vi "Dashboard Main.vi"() -> ()   [LabVIEW 2018]
uses:
  <vilib>/Utility/miscctls.llb/LVRowAndColumnTypeDef.ctl
  <vilib>/event_ctls.llb/eventvkey.ctl
  <vilib>/Rock Robotics/Network Tables/NT Read Numeric Array.vi
  <vilib>/Rock Robotics/Network Tables/NT Read Boolean.vi
  <vilib>/Rock Robotics/Network Tables/NT Write Boolean.vi
  <vilib>/Rock Robotics/WPI/Dashboard/WPI_DashboardLogging Global.vi
  <vilib>/Utility/xml.llb/Read From XML File(array).vi
  <vilib>/Utility/xml.llb/Write to XML File(string).vi
  <vilib>/vision/NI_Vision_Development_Module.lvlib
panel:
  out "Camera Image1":T1(plugin-control)
  out "Camera Image Right":T1(plugin-control)
  in  "Camera Settings Right":T2={"Frame Rate"=30, "Compression"=30, "Size"=1, "DB Camera Config"=FALSE} {"Frame Rate" scale=1.0..30.0; "Compression" scale=100.0..-1.0; "Size" items=["640x480", "320x240", "160x120"]}
  in  "Camera Name Right":string(combo)="No Camera Selection"
  in  "TCP":refnum<k5>
  in  "Rec Mode":enum32{"Stop", "Record", "Playback"}(radio)
  out "Robot IP":string
  out "Image Message":string="Timeout in Camera Communications"
  in  "Dashboard Tab":T3(tab)=enum."TeleOp"
  in  "CheckList":i32(listbox)
  out "Ret_CARGO Center":bool
  out "Elevator_Motor_Failure_2":bool
  out "Elevator_Stall":bool
  out "Range_Color_Front-Right":u32(colorbox)
  in  "Right":bool
  in  "Reticule":T4(ring)
  in  "Save":bool
  in  "Up":bool
  in  "Down":bool
  in  "Left":bool
  out "Ret_HATCH Right":bool
  out "Ret_HATCH Left":bool
  out "Ret_CARGO Right":bool
  out "Ret_CARGO Left":bool
  out "Out_Of_Time":bool caption="Mode_Butterfly"
  out "Match Time(s)":sgl
  out "Intake_In":bool caption="Mode_Butterfly"
  in  "Climb_Safety":bool
  out "Master_Caution":bool caption="Mode_Butterfly"
  out "Climb_Sequence":string
  out "Range_to_Target (R)":i16(slide)=-100 scale=-10.0..-50.0
  out "Range_to_Target (L)":i16(slide)=-100 scale=-50.0..-10.0
  out "Tilt_Interlock":bool
  out "Battery_Critical":bool
  out "Battery_Voltage":dbl(slide) scale=11.0..13.0
  out "COM_Warning":bool
  out "Elevator_Moving":bool caption="Mode_Butterfly"
  out "Range_Color_Back":u32(colorbox)
  out "Range_Color_Front-Left":u32(colorbox)
  out "Range_Color_Right":u32(colorbox)
  out "Range_Color_Left":u32(colorbox)
  out "Hatch_Ship_Light":bool
  out "Hatch_Rocket_1_Light":bool
  out "Hatch_Ground_Light":bool
  out "Hatch_Feeder_Light":bool
  out "Hatch_Rocket_2_Light":bool
  out "Hatch_Rocket_3_Light":bool
  out "Pressure_Visualize":dbl(slide) scale=0.0..120.0
  out "Autopilot":bool caption="Mode_Butterfly"
  in  "Master_Safety_Override_1":bool
  in  "Master_Safety_Override_2":bool
  out "Climb_Light":bool
  out "At Climb_Height":bool caption="Mode_Butterfly"
  out "PTO_Engaged":bool caption="Mode_Butterfly"
  in  "Climb":bool
  out "Mode_Butterfly":bool
  out "Compressor_On":bool
  out "Hatch_Ejection_State":bool caption="Mode_Butterfly"
  out "Elevator_Brake_State":bool
  out "Mode_Shift":bool caption="Mode_Butterfly"
  out "Capture_Cargo":bool caption="Mode_Butterfly"
  out "Capture_Hatch":bool caption="Mode_Butterfly"
  out "Right Feed":T1(plugin-control)
  in  "Hatch_Ground":bool
  in  "Hatch_Feeder":bool
  in  "Hatch_Rocket_2":bool
  in  "Hatch_Rocket_1":bool
  in  "Hatch_Ship":bool
  in  "Hatch_Rocket_3":bool
  out "Elevator_Stow_Light":bool
  in  "Elevator_Stow":bool
  out "Cargo_Ground_Light":bool
  out "Cargo_Feeder_Light":bool
  out "Cargo_Ship_Light":bool
  out "Cargo_Rocket_3_Light":bool
  in  "Cargo_Ground":bool
  in  "Cargo_Feeder":bool
  out "Cargo_Rocket_2_Light":bool
  out "Cargo_Rocket_1_Light":bool
  in  "Cargo_Ship":bool
  in  "Cargo_Rocket_1":bool
  in  "Cargo_Rocket_2":bool
  in  "Cargo_Rocket_3":bool
  out "State_Conflict":bool caption="Mode_Butterfly"
  out "Left Feed":T1(plugin-control)
  out "Elevator_Pos_Visual":dbl(slide) scale=34.5..89.0
  in  "Vision_Target_L_R":bool
  out "Elevator_Goal_Visual":dbl(slide) scale=34.5..89.0
  out "Elevator_Power":dbl(knob) scale=-1.0..1.0
  in  "Climb_Level":u8(slide)=1 scale=0.0..2.0
  in  "Driver Profile":u16(ring) items=["N/A"]
  out "E1 Warning":bool
  out "E2 Warning":bool
  out "E3 Warning":bool
  out "Elevator_3_Current":dbl format="%.1g"
  out "Elevator_2_Current":dbl format="%.1g"
  out "Elevator_1_Current":dbl format="%.1g"
  out "Slow_Loop":bool
  in  "Camera Settings 2":T2={"Frame Rate"=20, "Compression"=60, "Size"=1, "DB Camera Config"=FALSE} {"Size" items=["640x480", "320x240", "160x120"]}
  in  "Elevator_Kf_1":dbl(slide)=0.16 min=0.0 max=1.0 scale=0.0..1.0
  in  "Elevator_Kf_2":dbl(slide)=0.16 min=0.0 max=1.0 scale=0.0..1.0
  in  "Elevator_Kf_3":dbl(slide) min=0.0 max=1.0 scale=0.0..1.0
  in  "Select Auto":string(combo)="Select Autonomous ..."
  out "Camera Perf":string
  in  "Elevator_Kf_Climb":dbl(slide)=0.1 min=0.0 max=1.0 scale=0.0..1.0
  out "Control Loop Time (ms)":u32
  in  "Vacuum_Pump":dbl(slide)=0.6 min=0.0 max=1.0 scale=0.0..1.0
  out "Range_Right":dbl format="%.1g"
  in  "Elevator_Manual":bool
  in  "Drive_Encoder_Reset":bool
  out "Right_Drive_Pos":dbl
  out "Left_Drive_Pos":dbl
  out "Range_Left":dbl format="%.1g"
  out "Range_Front-Left":dbl format="%.1g"
  out "Range_Front-Right":dbl format="%.1g"
  out "Left_Drive_Vel":dbl format="%.1g"
  out "Right_Drive_Vel":dbl format="%.1g"
  out "Elevator_Pos":dbl format="%.1g"
  out "Range_Back":dbl
  out "Tank_Pressure":dbl
  in  "Super_Test_Mode":bool
  out "Ground_Height":dbl format="%.1g"
  in  "Overclock":bool=TRUE
  in  "Reinit_Stow_Vacuum":bool
  in  "LimeLight_Override":bool
  out "Elevator_Encoder_Malfunction":bool
  in  "Warning Time (s)":dbl=30.0
  out "Elevator_Motor_Failure":bool
  out "Robot_On_Ground":bool=TRUE
  out "Robot_Off_Ground":bool
  out "Check_Limit_Switch":bool
  in  "Tilt_Safety_Override":bool
  in  "Defense_Driving":bool
  out "NT Connection":bool
  out "Mode":T5(ring)=enum."Auto Disabled"
  out "Right Camera Perf":cluster{"Bandwidth (Mbps)":dbl, "FPS":dbl}
  in  "Test Slider":dbl(slide) scale=0.0..100.0 scale format="%#_3g"
  in  "On/Off":bool caption="Solenoid"
  in  "Test Name":u16(ring) items=["Select the test to run..."]
  in  "Test Tree":string(tree)
  in  "Motor":cluster{"Value":dbl, "Enable":bool} {"Value" scale=-1.0..1.0 scale format="%#_3g"}
  out "Progress":T6 {"Test Progress" scale=0.0..100.0}
  in  "Rev/Fwd":cluster{"Forward":bool, "Reverse":bool}
  in  "Test Ring":u16(ring) items=["Monochrome", "Color"]
  out "Cmd Status":string
  in  "Execute Command":bool
  in  "Command Params":string[][](table)
  in  "Command Selection":i32(listbox)
  out "Tree":string(tree)
  out "Background":bool
  in  "Camera Name":string(combo)="IMAQdx:Microsoft LifeCam"
  # "HW"
  # "11"
  # "13"
  # "Tina"
  # "Control Loop (ms)"
  # "Elevator Feed Forward Coefficients"
  # "Drive Wheel Velocities (ft/s)"
  # "Manual Elevator Override"
  # "Tilt Interlock Off"
  # "Wide-Cam Override"
  # "Reinit.  Vacuum in Stow"
  # "Super Test Mode"
  # "Elevator Position (in)"
  # "Prox Sensors (in)"
  # "Auto Elevator"
  # "Safe"
  # "Vacuum \nPump Power"
  # "Normal"
  # "Normal"
  # "Safe"
  # "Stage 2"
  # "Stage 3"
  # "Climb"
  # "Ground Height (in)"
  # "Elevator Motor Currents (A)"
  # "On \nGround"
  # "Off\nGround"
  # "E1"
  # "E2"
  # "E3"
  # "Match End Warning (s)"
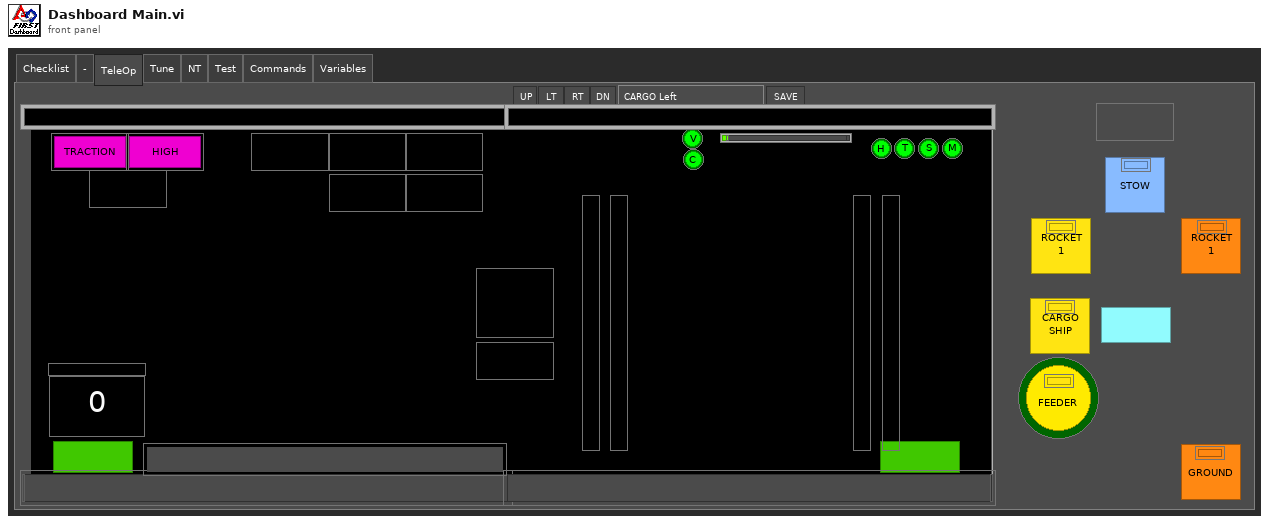
[diagram p1: front panel]
types:
  T1 = typedef "IMAQ Image.ctl" = refnum<image>
  T2 = cluster{"Frame Rate":i32, "Compression":i32, "Size":u16, "DB Camera Config":bool}
  T3 = enum32{"Checklist", "-", "TeleOp", "Tune", "NT", "Test", "Commands", "Variables"}
  T4 = enum16{"CARGO Left", "CARGO Right", "HATCH Left", "HATCH Right", "CARGO Center"}
  T5 = enum8{"Tele-Op Disabled", "Tele-Op Enabled", "Auto Disabled", "Auto Enabled", "Test Disabled", "Test Enabled", "Disconnected", "No Code", "E-Stop"}
  T6 = cluster{"Test Progress":u8, "Test Progress Text":string}
  T7 = cluster{"Save Path":path, "Interval (s)":dbl, "Keep":i32}
  T8 = enum32{"Drive", "Camera", "Basic", "Custom", "Test", "Commands", "Checklist", "Variables"}
  T9 = typedef "Image Type" = u32
  T10 = cluster{"IDs":cluster{"RPC field ID":u16, "Unique ID":u16}, "String":string}
  T11 = cluster{"Camera Image1":refnum<vi>, "Dashboard Tab":refnum<vi>, "Background":refnum<vi>, "Rec Mode":refnum<vi>, "Test Slider":refnum<vi>, "On/Off ":refnum<vi>, "Test Ring":refnum<vi>, "Rev/Fwd":refnum<vi>, "Test Name":refnum<vi>, "Motor":refnum<vi>, "Progress":refnum<vi>, "CheckList":refnum<vi>, "Tree":refnum<vi>, "Test Tree":refnum<vi>, "Command Params":refnum<vi>, "Command Selection":refnum<vi>, "Execute Command":refnum<vi>, "Cmd Status":refnum<vi>, "Camera Settings 2":refnum<vi>, "Camera Name":refnum<vi>, "Camera Perf":refnum<vi>, "Camera Settings Right":refnum<vi>, "Camera Name Right":refnum<vi>, "Camera Image Right":refnum<vi>}
  T12 = cluster{"Global Rectangle":i32[], "Contours":cluster{"Contour Type":u32, "ROI Type":u32, "Points":i32[]}[]}
  T13 = cluster{string, string, "Saved DB Images Info":cluster{"Save Path":path, "Interval (s)":dbl, "Keep":i32}}
  T14 = cluster{"Error Strings":string, "Disable Counts":cluster{u16, u16}, "Rail Faults":cluster{u16, u16, u16}, "Robot IP":string, "DB Mode":u8, "Event Info":cluster{"Name":string, "Type":u8, "Number":u16, "Replay":u8}}
  T15 = cluster{"Storage":cluster{"Disk Free":u64, "RAM Block":u32, "RAM free":u32}, "CPU Utilization":cluster{"CPU % ISR":sgl, "CPU % Time Crit":sgl, "CPU % Timed Str":sgl, "CPU % High":sgl, "CPU % Above":sgl, "CPU % Normal":sgl, "CPU % Low":sgl}, "CAN":cluster{"% Bus Utilization":sgl, "Bus Off Cnt":u32, "TX_FIFO Full Cnt":u32, "Receive Error Cnt":u8, "Transmit Error Cnt":u8}, "HID":cluster{"HID Outputs":u32, "Rumble Low":u16, "Rumble High":u16}[]}
  T16 = cluster{"Status bits":cluster{"Test Mode":bool, "Autonomous":bool, "Enabled":bool, "Code Start":bool, "Brownout":bool, "Reserved 2":bool, "Reserved 3":bool, "E-Stop":bool}, "Code Trace":cluster{"Disabled":bool, "TeleOp":bool, "Auto":bool, "Test":bool}, "Controller Type":enum16{"unknown", "cRIO", "roboRio"}, "Code?":enum16{"unknown", "noCode", "code"}, "Battery V":dbl}
  T17 = cluster{"Control Bits":cluster{"TestMode":bool, "Autonomous":bool, "Enabled":bool, "FMS Present":bool, bool, bool, bool, "E-Stop":bool}, "Team Station ":u8, "Countdown":sgl, "Joystick Values":cluster{"Axes":dbl[], "Buttons":bool[], "POVs":i16[]}[]}
  T18 = cluster{"Axes":dbl[], "Buttons":bool[], "POVs":i16[]}[]
  T19 = cluster{"Axes":dbl[], "Buttons":bool[], "POVs":i16[]}
  T20 = cluster{"Operation":enum16{"Update", "Clear"}, "Color Box":u32}[]
  T21 = typedef "eventvkey.ctl" = enum16{"ASCII", "Enter", "Return", "Shift", "Ctrl", "Alt", "Cmd", "Opt", "Caps", "NumLock", "Clear", "Break", "Up", "Down", "Left", "Right", "Insert", "Delete", "Home", "End", "PageUp", "PageDown", "Escape", "Help", "Pause", "ScrollLock", "F1", "F2", "F3", "F4", "F5", "F6", "F7", "F8", "F9", "F10", "F11", "F12", "F13", "F14", "F15", "F16", "F17", "F18", "F19", "F20", "F21", "F22", "F23", "F24", "Play", "VolumeUp", "VolumeDown", "Mute", "Two Byte Char"}
  T22 = cluster{"Image Size":bool, "Image Type":bool, "Pixel Value":bool, "ROI Information":bool, "Zoom Factor":bool}
  T23 = cluster{"Operation":enum16{"Update", "Clear"}, "Color Box":u32}
  T24 = typedef "LVRowAndColumnTypeDef.ctl" = cluster{"Row":i32, "Column":i32}
  T25 = cluster{"Shift":bool, "Ctrl":bool, "Alt":bool, "Cmd":bool, "Opt":bool}
  T26 = cluster{"Ret_CARGO Left":refnum<vi>, "Ret_CARGO Right":refnum<vi>, "Ret_HATCH Left":refnum<vi>, "Ret_HATCH Right":refnum<vi>, "Ret_CARGO Center":refnum<vi>}
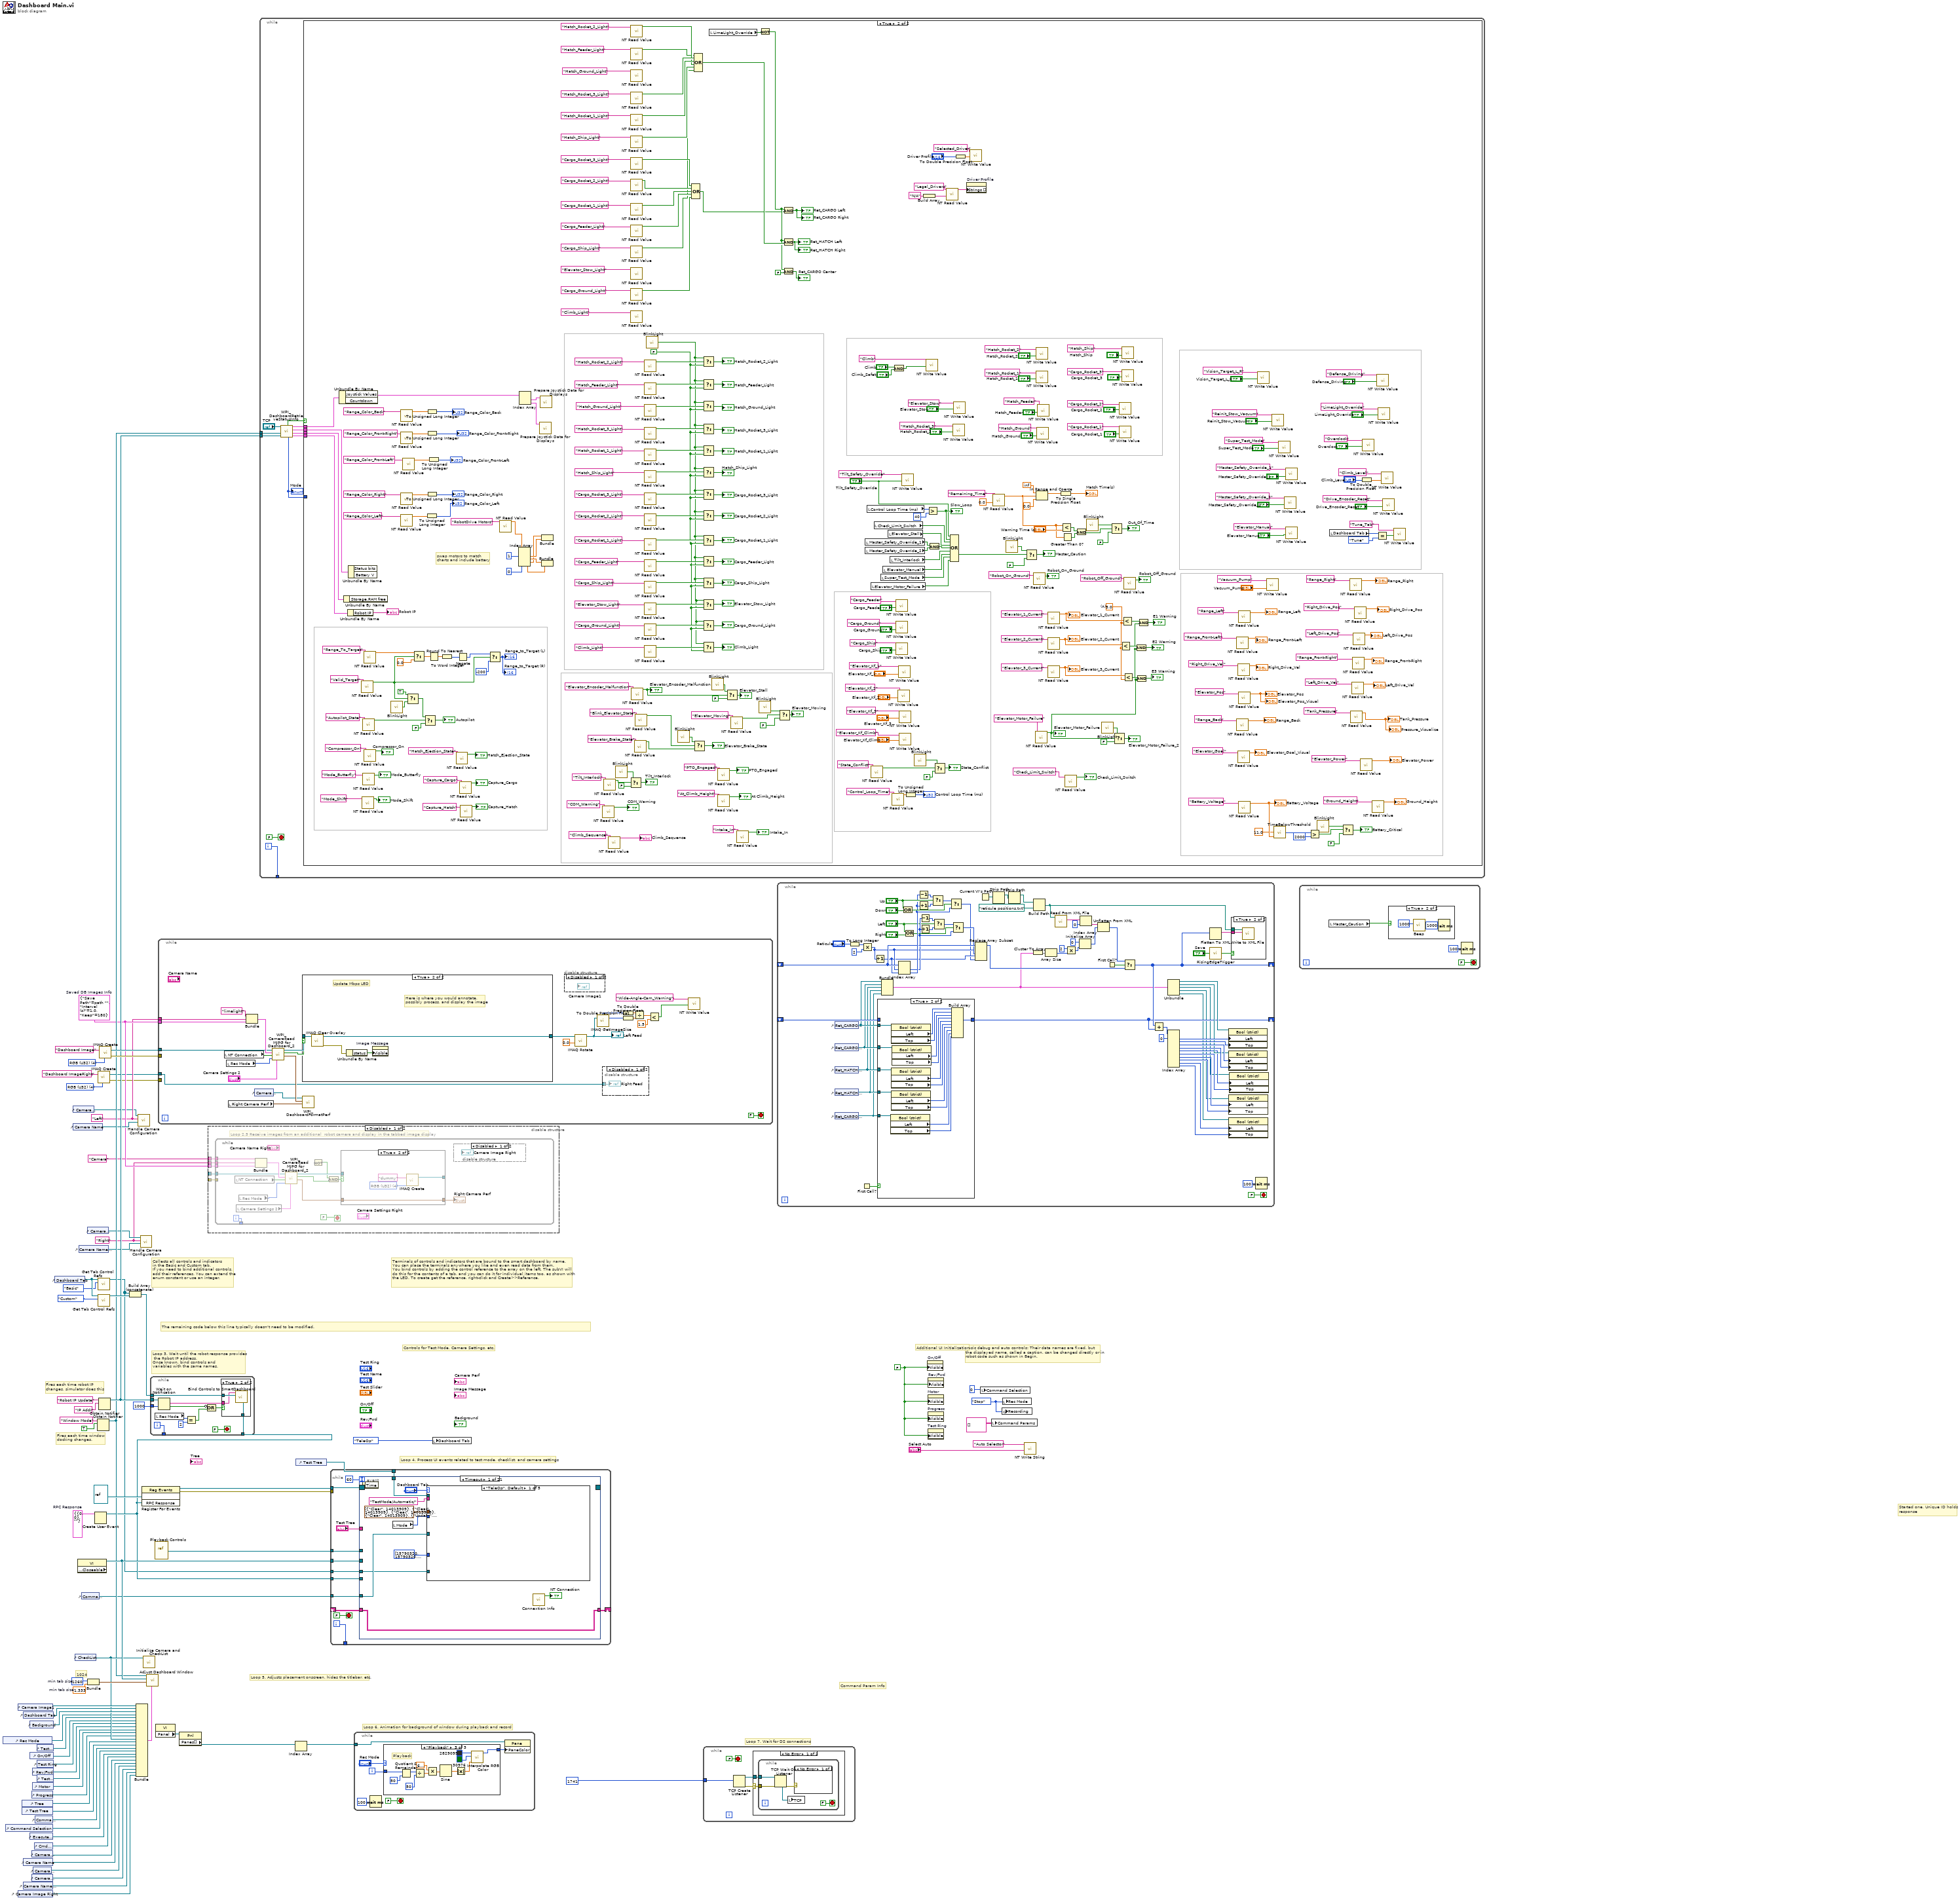
[diagram p0: block diagram]
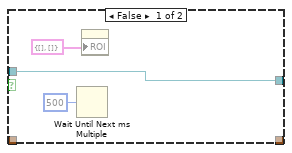
[diagram p6: hidden frame]
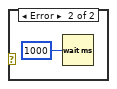
[diagram p8: hidden frame]
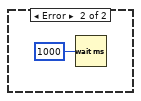
[diagram p9: hidden frame]
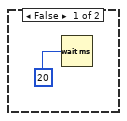
[diagram p10: hidden frame]
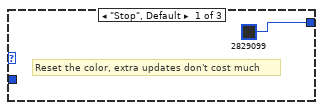
[diagram p11: hidden frame]
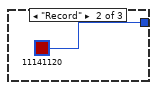
[diagram p12: hidden frame]
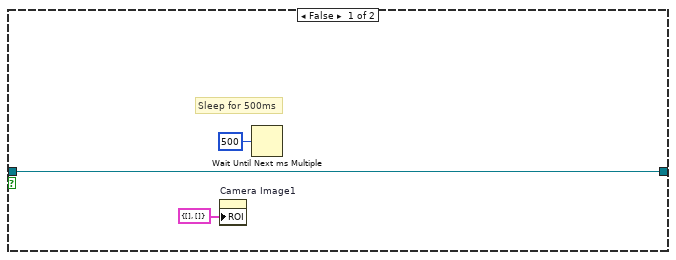
[diagram p16: hidden frame]
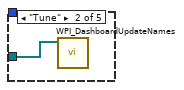
[diagram p17: hidden frame]
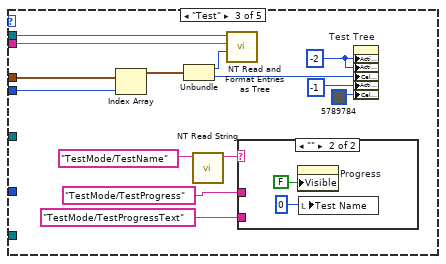
[diagram p18: hidden frame]
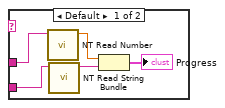
[diagram p19: hidden frame]
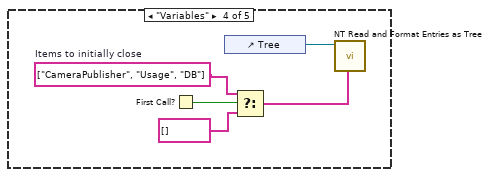
[diagram p20: hidden frame]
diagram:
  w8 = T7 {"Save Path"=path "", "Interval (s)"=1.0, "Keep"=180}  # Saved DB Images Info
  w7 = "Right"
  w6 = "Left"
  w16 = T9 4 items=["Grayscale (U8)", "Grayscale (I16)", "Grayscale (SGL)", "Complex (CSG)", "RGB (U32)", "HSL (U32)", "RGB (U64)"] ("Image Type")
  w30 = T10 {"IDs"={"RPC field ID"=0, "Unique ID"=0}, "String"=""}  # RPC Response
  w53 = 1260  # min tab size
  w52 = 1.333  # min tab size
  w60 = enum32{"Stop", "Record", "Playback"}."Stop" ("Rec Mode")
  w37 = FALSE ("Visible")
  w77 = T9 4 items=["Grayscale (U8)", "Grayscale (I16)", "Grayscale (SGL)", "Complex (CSG)", "RGB (U32)", "HSL (U32)", "RGB (U64)"] ("Image Type")
  # "1024"
  # "Command Param Info"
  # "Started one, Unique ID holds\nresponse"
  # "Loop 7. Wait for DS connections"
  # "Basic debug and auto controls: Their data names are fixed, but\nthe displayed name, called a caption, can be changed directly or in\nrobot code such as shown in Begin."
  # "Controls for Test Mode, Camera Settings, etc."
  # "Additional UI Initialization"
  # "Loop 6. Animation for background of window during playback and record"
  # "Fires each time robot IP\nchanges, simulator does this"
  # "Fires each time window\ndocking changes."
  # "Collects all controls and indicators\nin the Basic and Custom tab.\nIf you need to bind additional controls,\nadd their references. You can extend the\nenum constant or use an integer."
  # "The remaining code below this line typically doesn't need to be modified."
  # "Loop 4. Process UI events related to test mode, checklist, and camera settings"
  # "Terminals of controls and indicators that are bound to the smart dashboard by name.\nYou can place the terminals anywhere you like and even read data from them.\nYou bind controls by adding the control reference to the array on the left. The subVI will\ndo this for the contents of a tab, and you can do it for individual items too, as shown with\nthe LED. To create get the reference, right-click and Create>>Reference."
  # "Loop 3. Wait until the robot response provides\n the Robot IP address.\nOnce known, bind controls and\nvariables with the same names."
  # "Loop 5. Adjusts placement onscreen, hides the titlebar, etc."
  n1 = control-ref of="Rec Mode"() -> (w43:refnum<vi>)
  n2 = control-ref of="Command Selection"() -> (w29:refnum<vi>)
  n3 = control-ref of="Camera Image Right"() -> (w11:refnum<vi>)
  n4 = control-ref of="Camera Image1"() -> (w55:refnum<vi>)
  n5 = control-ref of="Tree"() -> (w47:refnum<vi>)
  n6 = control-ref of="Test Tree"() -> (w46:refnum<vi>)
  n7 = control-ref of="Dashboard Tab"() -> (w54:refnum<vi>)
  n8 = control-ref of="Camera Name"() -> (w22:refnum<vi>)
  n9 = control-ref of="Camera Name Right"() -> (w12:refnum<vi>)
  n10 = control-ref of="Execute Command"() -> (w31:refnum<vi>)
  n11 = control-ref of="Background"() -> (w50:refnum<vi>)
  n12 = control-ref of="On/Off"() -> (w41:refnum<vi>)
  n13 = control-ref of="Progress"() -> (w38:refnum<vi>)
  n14 = control-ref of="Camera Settings 2"() -> (w3:refnum<vi>)
  n15 = control-ref of="Camera Settings Right"() -> (w13:refnum<vi>)
  n16 = control-ref of="Rev/Fwd"() -> (w39:refnum<vi>)
  n17 = control-ref of="Motor"() -> (w44:refnum<vi>)
  n18 = control-ref of="Camera Perf"() -> (w21:refnum<vi>)
  n19 = control-ref of="Cmd Status"() -> (w25:refnum<vi>)
  n20 = control-ref of="Command Params"() -> (w32:refnum<vi>)
  n21 = control-ref of="Test Slider"() -> (w42:refnum<vi>)
  n22 = control-ref of="Test Ring"() -> (w40:refnum<vi>)
  n23 = control-ref of="Test Name"() -> (w45:refnum<vi>)
  n24 = control-ref of="Dashboard Tab"() -> (w58:refnum<vi>)
  n25 = control-ref of="Camera Name"() -> (w23:refnum<vi>)
  n26 = control-ref of="Camera Settings 2"() -> (w4:refnum<vi>)
  n27 = control-ref of="CheckList"() -> (w48:refnum<vi>)
  n28 = property class="VI" props=["Front Panel.Closeable"]() -> (reference out=w59:refnum<vi>)  [unwired: 2 in, 2 out]
  n29 = control-ref of="Camera Name Right"() -> (w14:refnum<vi>)
  n30 = control-ref of="Command Params"() -> (w24:refnum<vi>)
  n31 = control-ref of="Camera Settings Right"() -> (w15:refnum<vi>)
  n32 = Bundle("min tab size"=w53, "min tab size"=w52) -> (w51:cluster{"min tab size":i32, "min tab size":dbl})  [unwired: 1 in]
  n33 = Create User Event(user event datatype=w30) -> (user event=w26:refnum<user-event>)  [unwired: 1 in, 1 out]
  n34 = Obtain Notifier(name (unnamed)="Window Mode", notification data type=TRUE) -> (notifier out=w35:refnum<notifier>)  [unwired: 2 in, 2 out]
  n35 = call "IMAQ Create"("Image Name"="Dashboard ImageRight", "Image Type"=w16) -> ("New Image"=w2:T1, "error out"=w1:errorcluster)  [unwired: 2 in, 1 out]
  n36 = call <vilib>:"Get Tab Control Refs.vi"("Page Index"=T8."Basic" ("Dashboard Tab"), "TabControl in"=w58) -> ("ControlsOnPage"=w20:refnum<vi>[])  [unwired: 9 in]
  n37 = call <vilib>:"Get Tab Control Refs.vi"("Page Index"=T8."Custom" ("Dashboard Tab"), "TabControl in"=w58) -> ("ControlsOnPage"=w57:refnum<vi>[])  [unwired: 9 in]
  n38 = Obtain Notifier(name (unnamed)="Robot IP Update", notification data type="IP Addr" ("name (unnamed)")) -> (notifier out=w36:refnum<notifier>)  [unwired: 2 in, 2 out]
  n39 = call "IMAQ Create"("Image Name"="Dashboard Image", "Image Type"=w77) -> ("New Image"=w75:T1, "error out"=w74:errorcluster)  [unwired: 2 in, 1 out]
  n40 = Build Array (concatenate)(w20, w57) -> (w56:refnum<vi>[])
  n41 = Bundle("Camera Image1"=w55, "Dashboard Tab"=w54, "Background"=w50, "Rec Mode"=w43, "Test Slider"=w42, "On/Off"=w41, "Test Ring"=w40, "Rev/Fwd"=w39, "Test Name"=w45, "Motor"=w44, "Progress"=w38, "CheckList"=w48, "Tree"=w47, "Test Tree"=w46, "Command Params"=w32, "Command Selection"=w29, "Execute Command"=w31, "Cmd Status"=w25, "Camera Settings 2"=w3, "Camera Name"=w22, "Camera Perf"=w21, "Camera Settings Right"=w13, "Camera Name Right"=w12, "Camera Image Right"=w11) -> (w49:T11)  [unwired: 1 in]
  n42 = call "Handle Camera Configuration.vi"("CameraNameRef"=w23, "Display Name"=w6, "ClusterRef"=w4) -> ()  [unwired: 9 in]
  n43 = call "Handle Camera Configuration.vi"("CameraNameRef"=w14, "Display Name"=w7, "ClusterRef"=w15) -> ()  [unwired: 9 in]
  n44 = register-events(refnum<vi> refnum, w26) -> (reference out=w64:refnum<event-registration>, error out=w63:errorcluster)  [unwired: 2 in]
  n45 = call "Initialize Camera and CheckList.vi"("ListBox in"=w48) -> ()  [unwired: 11 in]
  n46 = call "Adjust Dashboard Window.vi"("Sizing Refnums"=w49, "Size Constraints"=w51, "VI"=w59, "WIn Mode"=w35) -> ()  [unwired: 8 in]
  n47 = while {
    tunnel: w56 -> [w89]
    tunnel: w36 -> [w87]
    tunnel: [w85] -> _
    tunnel: u32 1000 ("milliseconds to wait") -> [w84]
    tunnel: w26 -> [w78]
    i -> [w85]
    stop <- FALSE stop-if-true
    n48 = local read "Rec Mode"() -> (w80:enum32{"Stop", "Record", "Playback"})
    n49 = Wait on Notification(notifier=w87, timeout in ms (-1)=w84) -> (notification=w86:string, timed out?=w82:bool)  [unwired: 2 in, 2 out]
    n50 = Equal?(x=w80, y=u16 2 ("Rec Mode")) -> (x = y?=w81:bool)
    n51 = Compound Arithmetic op=OR(invert w82, w81) -> (w83:bool)
    n52 = case shown="True" w83 {
      tunnel: w89 -> [_ w92]
      tunnel: w86 -> [_ w91]
      tunnel: w78 -> [_ w90]
      frame False {
      }
      frame True {
        n53 = call <vilib>:"Bind Controls to SmartDashboard.vi"("RPC ref"=w90, "Bound Control Refs"=w92, "Server IP Address"=w91) -> ()  [unwired: 9 in]
      }
    }
  }
  n54 = vi-ref "Playback Controls.vi"() -> (w65:refnum<vi>)
  n55 = property class="VI"() -> ("Panel"=w67:refnum<vi>)  [unwired: 2 in, 2 out]
  n56 = while {
    tunnel: w75 -> [w105]
    tunnel: w74 -> [_]
    tunnel: w8 -> [w113]
    tunnel: w6 -> [w111]
    tunnel: w2 -> [w104]
    tunnel: w1 -> [_]
    stop <- FALSE stop-if-true
    n57 = local read "NT Connection"() -> (w114:bool)
    n58 = local read "Rec Mode"() -> (w115:enum32{"Stop", "Record", "Playback"})
    n59 = local read "Right Camera Perf"() -> (w109:cluster{"Bandwidth (Mbps)":dbl, "FPS":dbl})
    n60 = Bundle("limelight", w111, "Saved DB Images Info"=w113) -> (w112:T13)  [unwired: 1 in]
    n61 = control-ref of="Camera Perf"() -> (w108:refnum<vi>)
    n62 = call <vilib>:"WPI_CameraRead MJPG for Dashboard_2.vi"("Camera Settings"="Camera Settings 2", "Rec Mode"=w115, "NT Connection"=w114, "Capture Info"=w112, "Image in"=w105) -> ("perf info"=w110:cluster{"Bandwidth (Mbps)":dbl, "fps":dbl}, "Active"=w116:bool, "Image\\ out"=w117:T1)  [unwired: 4 in]
    n63 = case shown="True" w116 {
      tunnel: w117 -> [w121 w124]
      tunnel: [w121 w123] -> w103
      frame False {
        # "Sleep for 500ms"
        n64 = property on="Camera Image1" class="ImageControl"("ROI"=T12 {"Global Rectangle"=[], "Contours"=[]}) -> ()  [unwired: 2 in, 2 out]
        n65 = Wait Until Next ms Multiple(millisecond multiple=u32 500) -> ()  [unwired: 1 out]
      }
      frame True {
        # "Here is where you would annotate,\npossibly process, and display the image"
        # "Update Mbps LED"
        n66 = call "IMAQ Clear Overlay"("Image"=w124) -> ("error out"=w125:errorcluster, "Image Out"=w123:T1)  [unwired: 2 in, 7 out]
        n67 = Unbundle By Name(w125) -> ("status"=w126:bool)
        n68 = property on="Image Message" class="Str"("Visible"=w126) -> ()  [unwired: 2 in, 2 out]
      }
    }
    n69 = call <vilib>:"WPI_DashboardFormatPerf.vi"("Right Camera Perf"=w109, "Performance"=w110, "String in"=w108) -> ()  [unwired: 9 in]
    n70 = disable-structure shown="Disabled" {
      frame Disabled {
      }
      frame Enabled {
      }
    }
    n71 = call "IMAQ Rotate"("Angle (degrees)"=sgl 0.0, "Image Src"=w103) -> ("Image Dst Out"=w100:T1)  [unwired: 8 in, 1 out]
    "Left Feed" <- w100
    n72 = call "IMAQ GetImageSize"("Image"=w100) -> ("Y Resolution"=w96:i32, "X Resolution"=w97:i32)  [unwired: 3 in, 1 out]
    n73 = disable-structure shown="Disabled" {
      disable-tunnel: w104 -> [w119 _]
      frame Disabled {
        "Right Feed" <- w119
      }
      frame Enabled {
      }
    }
    n74 = To Double Precision Float(number=w97) -> (double precision float=w99:dbl)
    n75 = To Double Precision Float(number=w96) -> (double precision float=w98:dbl)
    n76 = Divide(x=w99, y=w98) -> (x/y=w95:dbl)
    n77 = Less?(x=w95, y=1.5) -> (x < y?=w93:bool)
    n78 = call-poly <vilib>:"NT Write Value.vi"("Boolean"=w93, "Name"="Wide-Angle-Cam_Warning") -> ()  [unwired: 9 in, 1 out]
  }
  n79 = property class="Pnl"(reference=w67) -> ("Panes[]"=w68:refnum<vi>[])  [unwired: 1 in, 2 out]
  n80 = disable-structure shown="Disabled" {
    disable-tunnel: _ -> [w131 _]
    disable-tunnel: _ -> [w130 _]
    disable-tunnel: w8 -> [w129 _]
    disable-tunnel: w7 -> [w128 _]
    disable-tunnel: "Camera" -> [w127 _]
    frame Disabled {
      # "Loop 2.5 Receive images from an additional  robot camera and display in the tabbed image display"
      n81 = while {
        tunnel: w131 -> [w136]
        tunnel: w130 -> [_]
        tunnel: [w145] -> _
        tunnel: w129 -> [w143]
        tunnel: w128 -> [w141]
        tunnel: w127 -> [w138]
        i -> [w145]
        stop <- FALSE stop-if-true
        n82 = local read "NT Connection"() -> (w144:bool)
        n83 = local read "Camera Settings 2"() -> (w137:T2)
        n84 = local read "Rec Mode"() -> (w148:enum32{"Stop", "Record", "Playback"})
        n85 = Bundle(w138, w141, "Saved DB Images Info"=w143) -> (w142:T13)  [unwired: 1 in]
        n86 = call <vilib>:"WPI_CameraRead MJPG for Dashboard_2.vi"("Camera Settings"=w137, "Rec Mode"=w148, "NT Connection"=w144, "Capture Info"=w142, "Image in"=w136) -> ("perf info"=w139:cluster{"Bandwidth (Mbps)":dbl, "fps":dbl}, "Active"=w135:bool, "Image\\ out"=w147:T1)  [unwired: 4 in]
        n87 = Not() -> (x=w134:bool, .not. x?=w132:bool)
        n88 = And(x=w132, y=w135) -> (x .and. y?=w133:bool)
        n89 = case shown="True" w133 {
          tunnel: w147 -> [w150 _]
          tunnel: [w150 w152] -> _
          tunnel: [_ w155] -> w140
          tunnel: w139 -> [_ w155]
          frame False {
            n90 = Wait Until Next ms Multiple(millisecond multiple=u32 500) -> ()  [unwired: 1 out]
            n91 = property on="Camera Image Right" class="ImageControl"("ROI"=T12 {"Global Rectangle"=[], "Contours"=[]}) -> ()  [unwired: 2 in, 2 out]
          }
          frame True {
            w154 = T9 4 items=["Grayscale (U8)", "Grayscale (I16)", "Grayscale (SGL)", "Complex (CSG)", "RGB (U32)", "HSL (U32)", "RGB (U64)", "Grayscale (U16)"] ("Image Type")
            n92 = call "IMAQ Create"("Image Name"="dummy", "Image Type"=w154) -> ("New Image"=w152:T1)  [unwired: 2 in, 2 out]
          }
        }
        "Right Camera Perf" <- w140
        n93 = disable-structure shown="Disabled" {
          frame Disabled {
          }
          frame Enabled {
          }
        }
      }
    }
    frame Enabled {
    }
  }
  n94 = while {
    tunnel: [w165] -> _
    tunnel: w36 -> [w159]
    tunnel: w35 -> [w156]
    i -> [w165]
    stop <- FALSE stop-if-true
    n95 = call <vilib>:"WPI_DashboardRetrieveStatusInfo.vi"("Binding Refnum"=w159, "Window Mode Notifier"=w156, "TCP Cnx"="TCP") -> ("Power and Errors"=w160:T14, "Robot Metrics"=w163:T15, "Status Info"=w164:T16, "Control Info"=w161:T17, "Robot Mode"=w158:T5, "Process?"=w162:bool)  [unwired: 3 in]
    "Mode" <- w158
    n96 = case shown="True" w162 {
      tunnel: w164 -> [_ w511]
      tunnel: w163 -> [_ w510]
      tunnel: w161 -> [_ w509]
      tunnel: w160 -> [_ w508]
      tunnel: w158 -> [_ _]
      frame False {
        n97 = Wait (ms)(milliseconds to wait=u32 20) -> ()  [unwired: 1 out]
      }
      frame True {
        w190 = 5.0  # (A)
        w351 = FALSE ("f")
        # "swap motors to match\ncharts and include battery"
        n98 = Unbundle By Name(w509) -> ("Joystick Values"=w501:T18)  [unwired: 1 out]
        n99 = Unbundle By Name(w510) -> ()  [unwired: 1 out]
        n100 = Unbundle By Name(w508) -> ("Robot IP"=→"Robot IP":string)
        n101 = Unbundle By Name(w511) -> ()  [unwired: 2 out]
        n102 = call-poly <vilib>:"NT Read Value.vi"("Name"="Valid_Target") -> ("Boolean"=w323:bool)  [unwired: 9 in, 1 out]
        n103 = call-poly <vilib>:"NT Read Value.vi"("Name"="Mode_Shift") -> ("Boolean"=→"Mode_Shift":bool)  [unwired: 9 in, 1 out]
        n104 = call-poly <vilib>:"NT Read Value.vi"("Name"="Mode_Butterfly") -> ("Boolean"=→"Mode_Butterfly":bool)  [unwired: 9 in, 1 out]
        n105 = call-poly <vilib>:"NT Read Value.vi"("Name"="Autopilot_State") -> ("Boolean"=w337:bool)  [unwired: 9 in, 1 out]
        n106 = call-poly <vilib>:"NT Read Value.vi"("Name"="Range_To_Target") -> ("Numeric"=w330:dbl)  [unwired: 9 in, 1 out]
        n107 = call-poly <vilib>:"NT Read Value.vi"("Name"="Compressor_On") -> ("Boolean"=→"Compressor_On":bool)  [unwired: 9 in, 1 out]
        n108 = call "BlinkLight.vi"() -> ("Blinked"=w332:bool)  [unwired: 1 in]
        n109 = call-poly <vilib>:"NT Read Value.vi"("Name"="Range_Color_Left") -> ("Numeric"=w488:dbl)  [unwired: 9 in, 1 out]
        n110 = call-poly <vilib>:"NT Read Value.vi"("Name"="Range_Color_Back") -> ("Numeric"=w494:dbl)  [unwired: 9 in, 1 out]
        n111 = call-poly <vilib>:"NT Read Value.vi"("Name"="Range_Color_Front-Right") -> ("Numeric"=w492:dbl)  [unwired: 9 in, 1 out]
        n112 = call-poly <vilib>:"NT Read Value.vi"("Name"="Range_Color_Right") -> ("Numeric"=w490:dbl)  [unwired: 9 in, 1 out]
        n113 = call-poly <vilib>:"NT Read Value.vi"("Name"="Range_Color_Front-Left") -> ("Numeric"=w442:dbl)  [unwired: 9 in, 1 out]
        n114 = Select(t=TRUE, s=w323, f=w332) -> (s? t:f=w335:bool)
        n115 = Select(t=w330, s=w323, f=0.0) -> (s? t:f=w328:dbl)
        n116 = Select(t=w335, s=w337, f=FALSE) -> (s? t:f=→"Autopilot":bool)
        n117 = To Unsigned Long Integer(number=w488) -> (unsigned 32bit integer=→"Range_Color_Left":u32)
        n118 = To Unsigned Long Integer(number=w494) -> (unsigned 32bit integer=→"Range_Color_Back":u32)
        n119 = To Unsigned Long Integer(number=w492) -> (unsigned 32bit integer=→"Range_Color_Front-Right":u32)
        n120 = To Unsigned Long Integer(number=w490) -> (unsigned 32bit integer=→"Range_Color_Right":u32)
        n121 = To Unsigned Long Integer(number=w442) -> (unsigned 32bit integer=→"Range_Color_Front-Left":u32)
        n122 = Round To Nearest(number=w328) -> (nearest integer value=w327:dbl)
        n123 = To Word Integer(number=w327) -> (16bit integer=w326:i16)
        n124 = call-poly <vilib>:"NT Read Value.vi"("Name"="Hatch_Ejection_State") -> ("Boolean"=→"Hatch_Ejection_State":bool)  [unwired: 9 in, 1 out]
        n125 = Negate(x=w326) -> (-x=w324:i16)
        n126 = call-poly <vilib>:"NT Read Value.vi"("Name"="Capture_Cargo") -> ("Boolean"=→"Capture_Cargo":bool)  [unwired: 9 in, 1 out]
        n127 = call-poly <vilib>:"NT Read Value.vi"("Name"="Capture_Hatch") -> ("Boolean"=→"Capture_Hatch":bool)  [unwired: 9 in, 1 out]
        n128 = Select(t=w324, s=w323, f=i16 -200) -> (s? t:f=→"Range_to_Target (L)" →"Range_to_Target (R)":i16)
        n129 = call-poly <vilib>:"NT Read Value.vi"("Name"="RobotDrive Motors") -> ("Numeric Array"=w497:dbl[])  [unwired: 9 in, 1 out]
        n130 = Index Array(array=w497, index #1=1, index #4=0) -> (element #1=w503:dbl, element #2=w504:dbl, element #3=w502:dbl, element #4=w507:dbl)  [unwired: 2 in]
        n131 = Index Array(array=w501) -> (element #1=w500:T19, element #2=w499:T19)  [unwired: 2 in]
        n132 = call "Prepare Joystick Data for Displays.vi"("Joystick Values"=w499) -> ()  [unwired: 8 in, 3 out]
        n133 = call "Prepare Joystick Data for Displays.vi"("Joystick Values"=w500) -> ()  [unwired: 8 in, 3 out]
        n134 = Bundle("Numeric"=w502, "Numeric"=w503) -> ()  [unwired: 1 in, 1 out]
        n135 = Bundle("Numeric"=w504, "Numeric"=w507) -> ()  [unwired: 1 in, 1 out]
        n136 = call-poly <vilib>:"NT Read Value.vi"("Name"="COM_Warning") -> ("Boolean"=→"COM_Warning":bool)  [unwired: 9 in, 1 out]
        n137 = call-poly <vilib>:"NT Read Value.vi"("Name"="Tilt_Interlock") -> ("Boolean"=w301:bool)  [unwired: 9 in, 1 out]
        n138 = call-poly <vilib>:"NT Read Value.vi"("Name"="Climb_Sequence") -> ("String"=→"Climb_Sequence":string)  [unwired: 9 in, 1 out]
        n139 = call "BlinkLight.vi"() -> ("Blinked"=w303:bool)  [unwired: 1 in]
        n140 = Select(t=w303, s=w301, f=FALSE) -> (s? t:f=→"Tilt_Interlock":bool)
        n141 = call-poly <vilib>:"NT Read Value.vi"("Name"="Hatch_Rocket_2_Light") -> ("Boolean"=w234:bool)  [unwired: 9 in, 1 out]
        n142 = call-poly <vilib>:"NT Read Value.vi"("Name"="Hatch_Feeder_Light") -> ("Boolean"=w232:bool)  [unwired: 9 in, 1 out]
        n143 = call-poly <vilib>:"NT Read Value.vi"("Name"="Hatch_Ground_Light") -> ()  [unwired: 9 in, 2 out]
        n144 = call-poly <vilib>:"NT Read Value.vi"("Name"="Hatch_Rocket_3_Light") -> ("Boolean"=w236:bool)  [unwired: 9 in, 1 out]
        n145 = call-poly <vilib>:"NT Read Value.vi"("Name"="Hatch_Rocket_1_Light") -> ("Boolean"=w235:bool)  [unwired: 9 in, 1 out]
        n146 = call-poly <vilib>:"NT Read Value.vi"("Name"="Hatch_Ship_Light") -> ("Boolean"=w233:bool)  [unwired: 9 in, 1 out]
        n147 = call-poly <vilib>:"NT Read Value.vi"("Name"="Cargo_Rocket_3_Light") -> ("Boolean"=w213:bool)  [unwired: 9 in, 1 out]
        n148 = call-poly <vilib>:"NT Read Value.vi"("Name"="Cargo_Rocket_2_Light") -> ("Boolean"=w212:bool)  [unwired: 9 in, 1 out]
        n149 = call-poly <vilib>:"NT Read Value.vi"("Name"="Cargo_Rocket_1_Light") -> ("Boolean"=w211:bool)  [unwired: 9 in, 1 out]
        n150 = call-poly <vilib>:"NT Read Value.vi"("Name"="Cargo_Feeder_Light") -> ("Boolean"=w210:bool)  [unwired: 9 in, 1 out]
        n151 = call-poly <vilib>:"NT Read Value.vi"("Name"="Cargo_Ship_Light") -> ("Boolean"=w176:bool)  [unwired: 9 in, 1 out]
        n152 = call-poly <vilib>:"NT Read Value.vi"("Name"="Elevator_Stow_Light") -> ()  [unwired: 9 in, 2 out]
        n153 = call-poly <vilib>:"NT Read Value.vi"("Name"="Cargo_Ground_Light") -> ("Boolean"=w175:bool)  [unwired: 9 in, 1 out]
        n154 = call-poly <vilib>:"NT Read Value.vi"("Name"="Climb_Light") -> ()  [unwired: 9 in, 2 out]
        n155 = call-poly <vilib>:"NT Read Value.vi"("Name"="Elevator_Encoder_Malfunction") -> ("Boolean"=w224:bool)  [unwired: 9 in, 1 out]
        "Elevator_Encoder_Malfunction" <- w224
        n156 = call-poly <vilib>:"NT Read Value.vi"("Name"="Elevator_Brake_State") -> ("Boolean"=w347:bool)  [unwired: 9 in, 1 out]
        n157 = call-poly <vilib>:"NT Read Value.vi"("Name"="Blink_Elevator_State") -> ("Boolean"=w346:bool)  [unwired: 9 in, 1 out]
        n158 = call-poly <vilib>:"NT Read Value.vi"("Name"="Hatch_Rocket_2_Light") -> ("Boolean"=w401:bool)  [unwired: 9 in, 1 out]
        n159 = call-poly <vilib>:"NT Read Value.vi"("Name"="Hatch_Feeder_Light") -> ("Boolean"=w399:bool)  [unwired: 9 in, 1 out]
        n160 = call-poly <vilib>:"NT Read Value.vi"("Name"="Hatch_Ground_Light") -> ("Boolean"=w398:bool)  [unwired: 9 in, 1 out]
        n161 = call-poly <vilib>:"NT Read Value.vi"("Name"="Hatch_Rocket_3_Light") -> ("Boolean"=w402:bool)  [unwired: 9 in, 1 out]
        n162 = call-poly <vilib>:"NT Read Value.vi"("Name"="Hatch_Rocket_1_Light") -> ("Boolean"=w400:bool)  [unwired: 9 in, 1 out]
        n163 = call-poly <vilib>:"NT Read Value.vi"("Name"="Hatch_Ship_Light") -> ("Boolean"=w397:bool)  [unwired: 9 in, 1 out]
        n164 = call-poly <vilib>:"NT Read Value.vi"("Name"="Cargo_Rocket_3_Light") -> ("Boolean"=w412:bool)  [unwired: 9 in, 1 out]
        n165 = call-poly <vilib>:"NT Read Value.vi"("Name"="Cargo_Rocket_2_Light") -> ("Boolean"=w411:bool)  [unwired: 9 in, 1 out]
        n166 = call-poly <vilib>:"NT Read Value.vi"("Name"="Cargo_Rocket_1_Light") -> ("Boolean"=w410:bool)  [unwired: 9 in, 1 out]
        n167 = call-poly <vilib>:"NT Read Value.vi"("Name"="Cargo_Feeder_Light") -> ("Boolean"=w409:bool)  [unwired: 9 in, 1 out]
        n168 = call-poly <vilib>:"NT Read Value.vi"("Name"="Cargo_Ship_Light") -> ("Boolean"=w415:bool)  [unwired: 9 in, 1 out]
        n169 = call-poly <vilib>:"NT Read Value.vi"("Name"="Elevator_Stow_Light") -> ("Boolean"=w365:bool)  [unwired: 9 in, 1 out]
        n170 = call-poly <vilib>:"NT Read Value.vi"("Name"="Cargo_Ground_Light") -> ("Boolean"=w413:bool)  [unwired: 9 in, 1 out]
        n171 = call-poly <vilib>:"NT Read Value.vi"("Name"="Climb_Light") -> ("Boolean"=w414:bool)  [unwired: 9 in, 1 out]
        n172 = call "BlinkLight.vi"() -> ("Blinked"=w350:bool)  [unwired: 1 in]
        n173 = call "BlinkLight.vi"() -> ("Blinked"=w345:bool)  [unwired: 1 in]
        n174 = Compound Arithmetic op=OR(w213, w212, w211, w210, w175) -> (w208:bool)
        n175 = Compound Arithmetic op=OR(w232, w236, w235, w234, w233, w176) -> (w231:bool)
        n176 = Select(t=w345, s=w346, f=w347) -> (s? t:f=→"Elevator_Brake_State":bool)
        n177 = Select(t=w350, s=w401, f=w351) -> (s? t:f=→"Hatch_Rocket_2_Light":bool)
        n178 = Select(t=w350, s=w399, f=w351) -> (s? t:f=→"Hatch_Feeder_Light":bool)
        n179 = Select(t=w350, s=w398, f=w351) -> (s? t:f=→"Hatch_Ground_Light":bool)
        n180 = Select(t=w350, s=w402, f=w351) -> (s? t:f=→"Hatch_Rocket_3_Light":bool)
        n181 = Select(t=w350, s=w400, f=w351) -> (s? t:f=→"Hatch_Rocket_1_Light":bool)
        n182 = Select(t=w350, s=w397, f=w351) -> (s? t:f=→"Hatch_Ship_Light":bool)
        n183 = Select(t=w350, s=w412, f=w351) -> (s? t:f=→"Cargo_Rocket_3_Light":bool)
        n184 = Select(t=w350, s=w411, f=w351) -> (s? t:f=→"Cargo_Rocket_2_Light":bool)
        n185 = Select(t=w350, s=w410, f=w351) -> (s? t:f=→"Cargo_Rocket_1_Light":bool)
        n186 = Select(t=w350, s=w409, f=w351) -> (s? t:f=→"Cargo_Feeder_Light":bool)
        n187 = Select(t=w350, s=w415, f=w351) -> (s? t:f=→"Cargo_Ship_Light":bool)
        n188 = Select(t=w350, s=w365, f=w351) -> (s? t:f=→"Elevator_Stow_Light":bool)
        n189 = Select(t=w350, s=w413, f=w351) -> (s? t:f=→"Cargo_Ground_Light":bool)
        n190 = Select(t=w350, s=w414, f=w351) -> (s? t:f=→"Climb_Light":bool)
        n191 = local read "LimeLight_Override"() -> (w239:bool)
        n192 = call "BlinkLight.vi"() -> ("Blinked"=w226:bool)  [unwired: 1 in]
        n193 = call-poly <vilib>:"NT Read Value.vi"("Name"="At_Climb_Height") -> ("Boolean"=→"At Climb_Height":bool)  [unwired: 9 in, 1 out]
        n194 = call-poly <vilib>:"NT Read Value.vi"("Name"="PTO_Engaged") -> ("Boolean"=→"PTO_Engaged":bool)  [unwired: 9 in, 1 out]
        n195 = Select(t=w226, s=w224, f=FALSE) -> (s? t:f=→"Elevator_Stall":bool)
        n196 = call-poly <vilib>:"NT Read Value.vi"("Name"="Elevator_Moving") -> ("Boolean"=w314:bool)  [unwired: 9 in, 1 out]
        n197 = call-poly <vilib>:"NT Read Value.vi"("Name"="Intake_In") -> ("Boolean"=→"Intake_In":bool)  [unwired: 9 in, 1 out]
        n198 = call "BlinkLight.vi"() -> ("Blinked"=w315:bool)  [unwired: 1 in]
        n199 = Not(x=w239) -> (.not. x?=w214:bool)
        n200 = Select(t=w315, s=w314, f=FALSE) -> (s? t:f=→"Elevator_Moving":bool)
        n201 = Compound Arithmetic op=AND(w214, w208) -> (→"Ret_CARGO Left" →"Ret_CARGO Right":bool)
        n202 = Compound Arithmetic op=AND(w214, w231) -> (→"Ret_HATCH Left" →"Ret_HATCH Right":bool)
        n203 = Compound Arithmetic op=AND(w214, FALSE ("value")) -> (→"Ret_CARGO Center":bool)
        n204 = local read "Master_Safety_Override_1"() -> (w281:bool)
        n205 = local read "Master_Safety_Override_2"() -> (w280:bool)
        n206 = local read "Control Loop Time (ms)"() -> (w275:u32)
        n207 = local read "Elevator_Motor_Failure"() -> (w207:bool)
        n208 = call-poly <vilib>:"NT Read Value.vi"("Name"="State_Conflict") -> ("Boolean"=w288:bool)  [unwired: 9 in, 1 out]
        n209 = local read "Check_Limit_Switch"() -> (w181:bool)
        n210 = local read "Super_Test_Mode"() -> (w276:bool)
        n211 = local read "Elevator_Manual"() -> (w277:bool)
        n212 = local read "Elevator_Stall"() -> (w279:bool)
        n213 = local read "Tilt_Interlock"() -> (w278:bool)
        n214 = call-poly <vilib>:"NT Read Value.vi"("Name"="Control_Loop_Time") -> ("Numeric"=w433:dbl)  [unwired: 9 in, 1 out]
        n215 = And(x="Climb", y="Climb_Safety") -> (x .and. y?=w320:bool)
        n216 = call-poly <vilib>:"NT Write Value.vi"("Boolean"="Cargo_Ship", "Name"="Cargo_Ship") -> ()  [unwired: 9 in, 1 out]
        n217 = call-poly <vilib>:"NT Write Value.vi"("Boolean"="Cargo_Feeder", "Name"="Cargo_Feeder") -> ()  [unwired: 9 in, 1 out]
        n218 = call-poly <vilib>:"NT Write Value.vi"("Boolean"="Cargo_Ground", "Name"="Cargo_Ground") -> ()  [unwired: 9 in, 1 out]
        n219 = call-poly <vilib>:"NT Write Value.vi"("Numeric"="Elevator_Kf_2", "Name"="Elevator_Kf_2") -> ()  [unwired: 9 in, 1 out]
        n220 = call-poly <vilib>:"NT Write Value.vi"("Numeric"="Elevator_Kf_1", "Name"="Elevator_Kf_1") -> ()  [unwired: 9 in, 1 out]
        n221 = call-poly <vilib>:"NT Write Value.vi"("Numeric"="Elevator_Kf_3", "Name"="Elevator_Kf_3") -> ()  [unwired: 9 in, 1 out]
        n222 = call-poly <vilib>:"NT Write Value.vi"("Numeric"="Elevator_Kf_Climb", "Name"="Elevator_Kf_Climb") -> ()  [unwired: 9 in, 1 out]
        n223 = call-poly <vilib>:"NT Write Value.vi"("Boolean"="Tilt_Safety_Override", "Name"="Tilt_Safety_Override") -> ()  [unwired: 9 in, 1 out]
        n224 = To Unsigned Long Integer(number=w433) -> (unsigned 32bit integer=→"Control Loop Time (ms)":u32)
        n225 = call "BlinkLight.vi"() -> ("Blinked"=w290:bool)  [unwired: 1 in]
        n226 = Build Array("N/A") -> (w169:string[])
        n227 = call-poly <vilib>:"NT Write Value.vi"("Boolean"=w320, "Name"="Climb") -> ()  [unwired: 9 in, 1 out]
        n228 = Greater?(x=w275, y=u32 40) -> (0:w182:bool)
        "Slow_Loop" <- w182
        n229 = And(x=w281, y=w280) -> (x .and. y?=w282:bool)
        n230 = Select(t=w290, s=w288, f=FALSE) -> (s? t:f=→"State_Conflict":bool)
        n231 = call-poly <vilib>:"NT Read Value.vi"("Default Value"=w169, "Name"="Legal_Drivers") -> ("String Array"=w171:string[])  [unwired: 8 in, 1 out]
        n232 = Compound Arithmetic op=OR("Tilt_Safety_Override", w182, w181, w279, w282, w278, w277, w276, w207) -> (w196:bool)
        n233 = call-poly <vilib>:"NT Write Value.vi"("Boolean"="Hatch_Rocket_3", "Name"="Hatch_Rocket_3") -> ()  [unwired: 9 in, 1 out]
        n234 = call-poly <vilib>:"NT Write Value.vi"("Boolean"="Elevator_Stow", "Name"="Elevator_Stow") -> ()  [unwired: 9 in, 1 out]
        n235 = To Double Precision Float(number="Driver Profile") -> (double precision float=w174:dbl)
        n236 = property on="Driver Profile" class="Ring (strict)"("Strings []"=w171) -> ()  [unwired: 2 in, 2 out]
        n237 = call-poly <vilib>:"NT Write Value.vi"("Numeric"=w174, "Name"="Selected_Driver") -> ()  [unwired: 9 in, 1 out]
        n238 = call-poly <vilib>:"NT Read Value.vi"("Default Value"=0.0, "Name"="Remaining_Time") -> ("Numeric"=w254:dbl)  [unwired: 8 in, 1 out]
        n239 = call "BlinkLight.vi"() -> ("Blinked"=w285:bool)  [unwired: 1 in]
        n240 = Select(t=w285, s=w196, f=FALSE) -> (s? t:f=→"Master_Caution":bool)
        n241 = call-poly <vilib>:"NT Read Value.vi"("Name"="Robot_On_Ground") -> ("Boolean"=→"Robot_On_Ground":bool)  [unwired: 9 in, 1 out]
        n242 = call-poly <vilib>:"NT Read Value.vi"("Name"="Elevator_Motor_Failure") -> ("Boolean"=w183:bool)  [unwired: 9 in, 1 out]
        "Elevator_Motor_Failure" <- w183
        n243 = In Range and Coerce(upper limit=inf, x=w254, lower limit=0.0) -> (coerced(x)=w257:dbl)  [unwired: 1 out]
        n244 = call-poly <vilib>:"NT Write Value.vi"("Boolean"="Hatch_Rocket_2", "Name"="Hatch_Rocket_2") -> ()  [unwired: 9 in, 1 out]
        n245 = call-poly <vilib>:"NT Write Value.vi"("Boolean"="Hatch_Rocket_1", "Name"="Hatch_Rocket_1") -> ()  [unwired: 9 in, 1 out]
        n246 = call-poly <vilib>:"NT Write Value.vi"("Boolean"="Hatch_Ground", "Name"="Hatch_Ground") -> ()  [unwired: 9 in, 1 out]
        n247 = call-poly <vilib>:"NT Write Value.vi"("Boolean"="Hatch_Feeder", "Name"="Hatch_Feeder") -> ()  [unwired: 9 in, 1 out]
        n248 = call-poly <vilib>:"NT Read Value.vi"("Name"="Elevator_1_Current") -> ("Numeric"=w193:dbl)  [unwired: 9 in, 1 out]
        "Elevator_1_Current" <- w193
        n249 = call-poly <vilib>:"NT Read Value.vi"("Name"="Elevator_2_Current") -> ("Numeric"=w192:dbl)  [unwired: 9 in, 1 out]
        "Elevator_2_Current" <- w192
        n250 = call-poly <vilib>:"NT Read Value.vi"("Name"="Elevator_3_Current") -> ("Numeric"=w191:dbl)  [unwired: 9 in, 1 out]
        "Elevator_3_Current" <- w191
        n251 = To Single Precision Float(number=w257) -> (single precision float=→"Match Time(s)":sgl)
        n252 = Less?(x=w254, y="Warning Time (s)") -> (x < y?=w260:bool)
        n253 = Greater Than 0?(x=w254) -> (x > 0?=w259:bool)
        n254 = call-poly <vilib>:"NT Read Value.vi"("Name"="Check_Limit_Switch") -> ("Boolean"=→"Check_Limit_Switch":bool)  [unwired: 9 in, 1 out]
        n255 = And(x=w260, y=w259) -> (x .and. y?=w258:bool)
        n256 = call "BlinkLight.vi"() -> ("Blinked"=w262:bool)  [unwired: 1 in]
        n257 = call "BlinkLight.vi"() -> ("Blinked"=w218:bool)  [unwired: 1 in]
        n258 = Select(t=w262, s=w258, f=FALSE) -> (s? t:f=→"Out_Of_Time":bool)
        n259 = Select(t=w218, s=w183, f=FALSE) -> (s? t:f=→"Elevator_Motor_Failure_2":bool)
        n260 = call-poly <vilib>:"NT Write Value.vi"("Boolean"="Cargo_Rocket_2", "Name"="Cargo_Rocket_2") -> ()  [unwired: 9 in, 1 out]
        n261 = call-poly <vilib>:"NT Write Value.vi"("Boolean"="Cargo_Rocket_1", "Name"="Cargo_Rocket_1") -> ()  [unwired: 9 in, 1 out]
        n262 = Less?(x=w192, y=w190) -> (x < y?=w188:bool)
        n263 = call-poly <vilib>:"NT Write Value.vi"("Boolean"="Cargo_Rocket_3", "Name"="Cargo_Rocket_3") -> ()  [unwired: 9 in, 1 out]
        n264 = Less?(x=w193, y=w190) -> (x < y?=w189:bool)
        n265 = call-poly <vilib>:"NT Write Value.vi"("Boolean"="Hatch_Ship", "Name"="Hatch_Ship") -> ()  [unwired: 9 in, 1 out]
        n266 = Less?(x=w191, y=w190) -> (x < y?=w187:bool)
        n267 = call-poly <vilib>:"NT Read Value.vi"("Name"="Robot_Off_Ground") -> ("Boolean"=→"Robot_Off_Ground":bool)  [unwired: 9 in, 1 out]
        n268 = Compound Arithmetic op=AND(w188, w183) -> (→"E2 Warning":bool)
        n269 = Compound Arithmetic op=AND(w187, w183) -> (→"E3 Warning":bool)
        n270 = Compound Arithmetic op=AND(w189, w183) -> (→"E1 Warning":bool)
        n271 = call-poly <vilib>:"NT Read Value.vi"("Name"="Range_Front-Left") -> ("Numeric"=→"Range_Front-Left":dbl)  [unwired: 9 in, 1 out]
        n272 = call-poly <vilib>:"NT Read Value.vi"("Name"="Range_Back") -> ("Numeric"=→"Range_Back":dbl)  [unwired: 9 in, 1 out]
        n273 = call-poly <vilib>:"NT Read Value.vi"("Name"="Right_Drive_Vel") -> ("Numeric"=→"Right_Drive_Vel":dbl)  [unwired: 9 in, 1 out]
        n274 = call-poly <vilib>:"NT Read Value.vi"("Name"="Elevator_Goal") -> ("Numeric"=→"Elevator_Goal_Visual":dbl)  [unwired: 9 in, 1 out]
        n275 = call-poly <vilib>:"NT Read Value.vi"("Name"="Range_Left") -> ("Numeric"=→"Range_Left":dbl)  [unwired: 9 in, 1 out]
        n276 = call-poly <vilib>:"NT Read Value.vi"("Name"="Elevator_Pos") -> ("Numeric"=→"Elevator_Pos" →"Elevator_Pos_Visual":dbl)  [unwired: 9 in, 1 out]
        n277 = call-poly <vilib>:"NT Read Value.vi"("Name"="Battery_Voltage") -> ("Numeric"=w200:dbl)  [unwired: 9 in, 1 out]
        "Battery_Voltage" <- w200
        n278 = call-poly <vilib>:"NT Write Value.vi"("Boolean"="Vision_Target_L_R", "Name"="Vision_Target_L_R") -> ()  [unwired: 9 in, 1 out]
        n279 = call-poly <vilib>:"NT Write Value.vi"("Numeric"="Vacuum_Pump", "Name"="Vacuum_Pump") -> ()  [unwired: 9 in, 1 out]
        n280 = call-poly <vilib>:"NT Write Value.vi"("Boolean"="Reinit_Stow_Vacuum", "Name"="Reinit_Stow_Vacuum") -> ()  [unwired: 9 in, 1 out]
        n281 = call "TimeBelowThreshold.vi"("Current Value"=w200, "Threshold"=11.0 ("y")) -> ("Time Below"=w198:u32)  [unwired: 3 in]
        n282 = call-poly <vilib>:"NT Write Value.vi"("Boolean"="Super_Test_Mode", "Name"="Super_Test_Mode") -> ()  [unwired: 9 in, 1 out]
        n283 = call-poly <vilib>:"NT Write Value.vi"("Boolean"="Master_Safety_Override_2", "Name"="Master_Safety_Override_2") -> ()  [unwired: 9 in, 1 out]
        n284 = call-poly <vilib>:"NT Write Value.vi"("Boolean"="Master_Safety_Override_1", "Name"="Master_Safety_Override_1") -> ()  [unwired: 9 in, 1 out]
        n285 = call-poly <vilib>:"NT Write Value.vi"("Boolean"="Elevator_Manual", "Name"="Elevator_Manual") -> ()  [unwired: 9 in, 1 out]
        n286 = Greater?(x=w198, y=u32 2000) -> (0:w305:bool)
        n287 = call "BlinkLight.vi"() -> ("Blinked"=w307:bool)  [unwired: 1 in]
        n288 = local read "Dashboard Tab"() -> (w344:T3)
        n289 = Select(t=w307, s=w305, f=FALSE) -> (s? t:f=→"Battery_Critical":bool)
        n290 = call-poly <vilib>:"NT Read Value.vi"("Name"="Range_Right") -> ("Numeric"=→"Range_Right":dbl)  [unwired: 9 in, 1 out]
        n291 = call-poly <vilib>:"NT Read Value.vi"("Name"="Tank_Pressure") -> ("Numeric"=→"Tank_Pressure" →"Pressure_Visualize":dbl)  [unwired: 9 in, 1 out]
        n292 = call-poly <vilib>:"NT Read Value.vi"("Name"="Left_Drive_Vel") -> ("Numeric"=→"Left_Drive_Vel":dbl)  [unwired: 9 in, 1 out]
        n293 = call-poly <vilib>:"NT Read Value.vi"("Name"="Range_Front-Right") -> ("Numeric"=→"Range_Front-Right":dbl)  [unwired: 9 in, 1 out]
        n294 = call-poly <vilib>:"NT Read Value.vi"("Name"="Left_Drive_Pos") -> ("Numeric"=→"Left_Drive_Pos":dbl)  [unwired: 9 in, 1 out]
        n295 = call-poly <vilib>:"NT Read Value.vi"("Name"="Right_Drive_Pos") -> ("Numeric"=→"Right_Drive_Pos":dbl)  [unwired: 9 in, 1 out]
        n296 = call-poly <vilib>:"NT Read Value.vi"("Name"="Elevator_Power") -> ("Numeric"=→"Elevator_Power":dbl)  [unwired: 9 in, 1 out]
        n297 = To Double Precision Float(number="Climb_Level") -> (double precision float=w205:dbl)
        n298 = call-poly <vilib>:"NT Write Value.vi"("Boolean"="Overclock", "Name"="Overclock") -> ()  [unwired: 9 in, 1 out]
        n299 = call-poly <vilib>:"NT Read Value.vi"("Name"="Ground_Height") -> ("Numeric"=→"Ground_Height":dbl)  [unwired: 9 in, 1 out]
        n300 = Equal?(x=w344, y=T3."Tune") -> (x = y?=w342:bool)
        n301 = call-poly <vilib>:"NT Write Value.vi"("Boolean"="Defense_Driving", "Name"="Defense_Driving") -> ()  [unwired: 9 in, 1 out]
        n302 = call-poly <vilib>:"NT Write Value.vi"("Boolean"="LimeLight_Override", "Name"="LimeLight_Override") -> ()  [unwired: 9 in, 1 out]
        n303 = call-poly <vilib>:"NT Write Value.vi"("Numeric"=w205, "Name"="Climb_Level") -> ()  [unwired: 9 in, 1 out]
        n304 = call-poly <vilib>:"NT Write Value.vi"("Boolean"="Drive_Encoder_Reset", "Name"="Drive_Encoder_Reset") -> ()  [unwired: 9 in, 1 out]
        n305 = call-poly <vilib>:"NT Write Value.vi"("Boolean"=w342, "Name"="Tune_Tab") -> ()  [unwired: 9 in, 1 out]
      }
    }
  }
  n306 = Index Array(array=w68) -> (element=w66:refnum<vi>)  [unwired: 1 in]
  n307 = control-ref of="Test Tree"() -> (w69:refnum<vi>)
  n308 = while {
    tunnel: [w521] -> _
    tunnel: w69 -> [w520]
    tunnel: w65 -> [w519]
    tunnel: w64 -> [w518]
    tunnel: w63 -> [_]
    tunnel: w59 -> [w517]
    tunnel: w26 -> [w516]
    tunnel: w24 -> [w515]
    shift-right: [w514] -> _
    shift-left: _ -> [w513]
    tunnel: w20 -> [w512]
    i -> [w521]
    stop <- FALSE stop-if-true
    n309 = event shown="[0] Timeout" {
      selector: w518 -> [_ _ _ _ _ _ _ _ _ _ _ _ _ _ _ _ _ _ _ _ _]
      dyn-events: [_ _ _ _ _ _ _ _ _ _ _ _ _ _ _ _ w781 _ _ _ _] -> _
      timeout: u32 60 ("milliseconds to wait") -> [_ _ _ _ _ _ _ _ _ _ _ _ _ _ _ _ _ _ _ _ _]
      tunnel: w520 -> [w533 _ _ _ _ _ _ _ _ _ _ _ _ _ _ _ _ _ _ _ _]
      tunnel: "Test Tree" -> [_ _ _ _ _ _ _ _ _ _ _ w748 w756 w758 w762 w770 _ _ _ _ _]
      tunnel: w519 -> [_ _ _ _ _ _ _ _ _ _ _ _ _ _ _ _ w783 _ w801 _ _]
      tunnel: w517 -> [_ _ _ _ _ _ _ _ _ _ _ _ _ _ _ _ w779 _ _ _ _]
      tunnel: w516 -> [_ _ _ _ _ _ _ _ _ _ _ _ _ _ _ _ w777 _ _ _ _]
      tunnel: w515 -> [w528 _ _ _ _ _ w699 _ _ _ _ _ _ _ _ _ _ _ _ _ _]
      tunnel: [w527 w576 w678 w683 w692 w696 w697 w706 w716 w723 w735 w747 w754 w757 w761 w769 w776 w796 w798 w802 w815] -> w514
      tunnel: w513 -> [w527 w576 w678 w683 w692 w696 w697 _ _ w723 w735 w747 w754 w757 w761 w769 w776 w796 w798 w802 w815]
      tunnel: w512 -> [w525 _ _ _ _ _ _ _ _ _ _ _ _ _ _ _ _ _ _ _ _]
      event Timeout {
        n310 = event-data() -> ()  [unwired: 1 in, 1 out]
        n311 = local read "Mode"() -> (w530:T5)
        n312 = case shown="\"TeleOp\", Default" "Dashboard Tab" {
          tunnel: w533 -> [_ _ w549 _ _]
          tunnel: "TestMode/Automatic/" ("Name Pattern") -> [_ _ w548 _ _]
          tunnel: T20 [{"Operation"=enum."Clear", "Color Box"=14013909}, {"Operation"=enum."Clear", "Color Box"=14013909}, {"Operation"=enum."Clear", "Color Box"=14013909}, {"Operation"=enum."Clear", "Color Box"=14013909}, {"Operation"=enum."Update", "Color Box"=14013909}, {"Operation"=enum."Update", "Color Box"=16777215}, {"Operation"=enum."Clear", "Color Box"=14013909}, {"Operation"=enum."Clear", "Color Box"=14013909}, {"Operation"=enum."Clear", "Color Box"=14013909}] -> [_ _ w541 _ w569]
          tunnel: w530 -> [_ _ w540 _ w568]
          tunnel: u32[] [15790320, 15790320, 15790320, 15790320, 16777215, 16777215, 15790320, 15790320, 15790320] -> [_ _ _ _ w574]
          tunnel: w528 -> [_ _ _ _ w562]
          tunnel: w525 -> [_ w535 _ _ _]
          frame "TeleOp", Default {
          }
          frame "Tune" {
            n313 = call <vilib>:"WPI_DashboardUpdateNames.vi"("Controls on Tab"=w535) -> ()  [unwired: 11 in]
          }
          frame "Test" {
            w547 = -2 ("Active Item:Row Number")
            n314 = Index Array(array=w541, index=w540) -> (element=w542:T23)
            n315 = Unbundle(w542) -> ("Operation"=w543:enum16{"Update", "Clear"}, "Color Box"=w544:u32)
            n316 = call <vilib>:"NT Read String.vi"("Name"="TestMode/TestName") -> ("String"=w538:string)  [unwired: 9 in, 1 out]
            n317 = call <vilib>:"NT Read and Format Entries as Tree.vi"("Operation"=w543, "Name Pattern"=w548, "Tree Refnum"=w549) -> ()  [unwired: 7 in, 2 out]
            n318 = case shown="\"\"" w538 {
              tunnel: "TestMode/TestProgress" ("Name") -> [w551 _]
              tunnel: "TestMode/TestProgressText" ("Name") -> [w550 _]
              frame Default {
                n319 = call <vilib>:"NT Read Number.vi"("Name"=w551) -> ("Numeric"=w552:dbl)  [unwired: 9 in, 1 out]
                n320 = call <vilib>:"NT Read String.vi"("Name"=w550) -> ("String"=w553:string)  [unwired: 9 in, 1 out]
                n321 = Bundle("Numeric"=w552, "String"=w553) -> (→"Progress":cluster{"Numeric":dbl, "String":string})  [unwired: 1 in]
              }
              frame "" {
                n322 = property on="Progress" class="Clust (strict)"("Visible"=FALSE) -> ()  [unwired: 2 in, 2 out]
                n323 = local write "Test Name"(u16 0) -> ()
              }
            }
            n324 = property on="Test Tree" class="Tree (strict)"("Active Item Row Number"=w547, "ActiveColNum"=w547, "CellBG"=w544, "Active Item Row Number"=-1 ("Active Item:Row Number"), "CellBG"=u32 5789784 ("Color Box")) -> ()  [unwired: 2 in, 2 out]
          }
          frame "Variables" {
            w559 = string[] ["CameraPublisher", "Usage", "DB"]  # Items to initially close
            n325 = First Call?() -> (First Call?: T/F=w560:bool)
            n326 = control-ref of="Tree"() -> (w561:refnum<vi>)
            n327 = Select(t=w559, s=w560, f=string[] []) -> (s? t:f=w557:string[])
            n328 = call <vilib>:"NT Read and Format Entries as Tree.vi"("Tags to  Close"=w557, "Tree Refnum"=w561) -> ()  [unwired: 8 in, 2 out]
          }
          frame "Commands" {
            w570 = u32 5789784 ("Color Box")
            w571 = T24 {"Row"=-1, "Column"=-2} ("Active Cell:Active Cell")
            w573 = T24 {"Row"=-2, "Column"=-2} ("Active Cell:Active Cell")
            n329 = Index Array(array=w574, index=w568) -> (element=w572:u32)
            n330 = Index Array(array=w569, index=w568) -> (element=w567:T23)
            n331 = Unbundle(w567) -> ("Operation"=w566:enum16{"Update", "Clear"})  [unwired: 1 out]
            n332 = local read "Command Selection"() -> (w565:i32)
            n333 = property on="Command Selection" class="MCListbox (strict)"("ActiveCell"=w573, "CellBG"=w572, "ActiveCell"=w571, "CellBG"=w570) -> ()  [unwired: 2 in, 2 out]
            n334 = call <vilib>:"WPI_DashboardUpdate RPC Info.vi"("Operation"=w566) -> ("update"=w564:bool, "commands"=w563:string[][])  [unwired: 9 in]
            n335 = property on="Command Selection" class="MCListbox (strict)"("ItemNames"=w563) -> ()  [unwired: 2 in, 2 out]
            n336 = property on="Command Params" class="Tbl (strict)"("Active Cell"=w573, "Cell BG Color"=w572, "Active Cell"=w571, "Cell BG Color"=w570) -> ()  [unwired: 2 in, 2 out]
            n337 = call <vilib>:"WPI_DashboardUpdate Command Params.vi"("Update"=w564, "NewVal"=w565, "Commands"=w563, "Param Tbl"=w562) -> ()  [unwired: 7 in, 1 out]
          }
        }
        n338 = call <vilib>:"Connextion Info.vi"() -> ("Connected"=→"NT Connection":bool)  [unwired: 10 in, 1 out]
      }
      event "Test Tree": Value Change {
        # "Show appropriate\ncontrols"
        n339 = event-data() -> ("CtlRef"=w579:refnum<vi>, "NewVal"=w577:string)  [unwired: 1 in]
        n340 = call <vilib>:"WPI_UtilitiesGetTreeIOName.vi"("NewVal"=w577, "TreeControl in"=w579) -> ("I/O Name"=w580:string)  [unwired: 9 in]
        n341 = case shown="\"Camera\"" w580 {
          selector: w580 -> [_ w587 _ w609 w618 _]
          tunnel: w577 -> [_ _ w606 w608 _ w625]
          tunnel: cluster{string[]}[] [{["640x480", "320x240", "160x120"]}, {["Auto", "Fixed indoor", "Fixed outdoor 1", "Fixed outdoor 2", "Fixed fluorescent 1", "Fixed fluorescent 2", "Hold current"]}, {["Auto", "Flicker-free 50 Hz", "Flicker-free 60 Hz", "Hold current"]}, {["None", "Prioritize frame rate", "Prioritize image quality"]}, {["Monochrome", "Color"]}] -> [_ _ _ _ _ w624]
          frame Default {
            w582 = FALSE ("Visible")
            w581 = FALSE ("Visible")
            n342 = property on="Motor" class="Clust (strict)"("Visible"=w581) -> ()  [unwired: 2 in, 2 out]
            n343 = property on="Test Ring" class="Ring (strict)"("Visible"=w581) -> ()  [unwired: 2 in, 2 out]
            n344 = property on="Rev/Fwd" class="Clust (strict)"("Visible"=w582) -> ()  [unwired: 2 in, 2 out]
            n345 = property on="On/Off" class="Bool (strict)"("Visible"=w582) -> ()  [unwired: 2 in, 2 out]
            n346 = property on="Test Slider" class="Slide (strict)"("Visible"=w582) -> ()  [unwired: 2 in, 2 out]
          }
          frame "Analog Out", "Motor", "PWM" {
            w588 = FALSE ("Visible")
            n347 = case shown="\"Analog Out\"" w587 {
              tunnel: [1.0 ("Value") -1.0 ("Value") 0.0 ("Value")] -> w586
              tunnel: [255.0 ("Value") 1.0 ("Value") 5.0 ("Value")] -> w585
              tunnel: [128.0 ("Value") 0.0 ("Value") 0.0 ("Value")] -> w584
              tunnel: [64.0 ("Value") 0.5 ("Value") 1.0 ("Value")] -> w583
              frame "PWM" {
              }
              frame "Motor", Default {
              }
              frame "Analog Out" {
              }
            }
            n348 = property on="Motor" class="Clust (strict)"("Visible"=TRUE) -> ()  [unwired: 2 in, 2 out]
            n349 = property on="Value" class="Slide (strict)"("Value"=w584, "Scale.Minimum"=w586, "Scale.Maximum"=w585, "Scale.Increment"=w583) -> ()  [unwired: 2 in, 2 out]
            n350 = property on="On/Off" class="Bool (strict)"("Visible"=w588) -> ()  [unwired: 2 in, 2 out]
            n351 = property on="Test Slider" class="Slide (strict)"("Visible"=w588) -> ()  [unwired: 2 in, 2 out]
            n352 = property on="Test Ring" class="Ring (strict)"("Visible"=w588) -> ()  [unwired: 2 in, 2 out]
            n353 = property on="Rev/Fwd" class="Clust (strict)"("Visible"=w588) -> ()  [unwired: 2 in, 2 out]
          }
          frame "Servo" {
            w604 = FALSE ("Visible")
            n354 = call <vilib>:"NT Read Number.vi"("Name"=w606) -> ("Numeric"=w605:dbl)  [unwired: 9 in, 1 out]
            n355 = property on="Test Slider" class="Slide (strict)"("Visible"=TRUE, "Scale.Maximum"=170.0 ("Scale.Range:Maximum")) -> ()  [unwired: 2 in, 2 out]
            n356 = local write "Test Slider"(w605) -> ()
            n357 = property on="Motor" class="Clust (strict)"("Visible"=w604) -> ()  [unwired: 2 in, 2 out]
            n358 = property on="Rev/Fwd" class="Clust (strict)"("Visible"=w604) -> ()  [unwired: 2 in, 2 out]
            n359 = property on="On/Off" class="Bool (strict)"("Visible"=w604) -> ()  [unwired: 2 in, 2 out]
            n360 = property on="Test Ring" class="Ring (strict)"("Visible"=w604) -> ()  [unwired: 2 in, 2 out]
          }
          frame "Relay", "Solenoid" {
            w607 = FALSE ("Visible")
            n361 = property on="Motor" class="Clust (strict)"("Visible"=w607) -> ()  [unwired: 2 in, 2 out]
            n362 = property on="Test Slider" class="Slide (strict)"("Visible"=w607) -> ()  [unwired: 2 in, 2 out]
            n363 = Search and Replace String(input string=w608, search string="/Value  **", replace string="/Direction") -> (result string=w614:string)  [unwired: 5 in, 3 out]
            n364 = property on="Test Ring" class="Ring (strict)"("Visible"=w607) -> ()  [unwired: 2 in, 2 out]
            n365 = call <vilib>:"NT Read String.vi"("Name"=w614) -> ("String"=w612:string)  [unwired: 9 in, 1 out]
            n366 = Equal?(x="Both directions", y=w612) -> (x = y?=w610:bool)
            n367 = Not(x=w610) -> (.not. x?=w611:bool)
            n368 = property on="Rev/Fwd" class="Clust (strict)"("Visible"=w610) -> ()  [unwired: 2 in, 2 out]
            n369 = property on="On/Off" class="Bool (strict)"("Visible"=w611, "Caption.Text"=w609) -> ()  [unwired: 2 in, 2 out]
          }
          frame "Compressor", "Digital Out" {
            w617 = FALSE ("Visible")
            # "Get direction and finish"
            n370 = property on="Motor" class="Clust (strict)"("Visible"=w617) -> ()  [unwired: 2 in, 2 out]
            n371 = property on="Test Slider" class="Slide (strict)"("Visible"=w617) -> ()  [unwired: 2 in, 2 out]
            n372 = property on="Test Ring" class="Ring (strict)"("Visible"=w617) -> ()  [unwired: 2 in, 2 out]
            n373 = property on="On/Off" class="Bool (strict)"("Visible"=TRUE, "Caption.Text"=w618) -> ()  [unwired: 2 in, 2 out]
            n374 = property on="Rev/Fwd" class="Clust (strict)"("Visible"=FALSE) -> ()  [unwired: 2 in, 2 out]
          }
          frame "Camera" {
            n375 = call <vilib>:"Get Last Path Segment.vi"("String in"=w625) -> ("String out"=w626:string)  [unwired: 10 in]
            n376 = property on="On/Off" class="Bool (strict)"("Visible"=FALSE) -> ()  [unwired: 2 in, 2 out]
            n377 = property on="Motor" class="Clust (strict)"("Visible"=FALSE) -> ()  [unwired: 2 in, 2 out]
            n378 = property on="Rev/Fwd" class="Clust (strict)"("Visible"=FALSE) -> ()  [unwired: 2 in, 2 out]
            n379 = case shown="\"White Balance  **\"" w626 {
              tunnel: w625 -> [w632 w641 w650 w659 w668 _ w674]
              tunnel: w624 -> [w630 w638 w647 w656 w665 _ _]
              frame "Size  **" {
                n380 = Index Array(array=w630) -> (element=w629:cluster{string[]})  [unwired: 1 in]
                n381 = call <vilib>:"NT Read String.vi"("Name"=w632) -> ("String"=w631:string)  [unwired: 9 in, 1 out]
                n382 = Unbundle(w629) -> (w627:string[])
                n383 = Match First String(2:w627, 3:w631) -> (0:w628:i32)  [unwired: 1 out]
                n384 = property on="Test Ring" class="Ring (strict)"("Value"=w628, "Strings []"=w627) -> ()  [unwired: 2 in, 2 out]
                n385 = property on="Test Ring" class="Ring (strict)"("Visible"=TRUE) -> ()  [unwired: 2 in, 2 out]
                n386 = property on="Test Slider" class="Slide (strict)"("Visible"=FALSE) -> ()  [unwired: 2 in, 2 out]
              }
              frame "White Balance  **" {
                n387 = Index Array(array=w638, index=1) -> (element=w639:cluster{string[]})
                n388 = call <vilib>:"NT Read String.vi"("Name"=w641) -> ("String"=w640:string)  [unwired: 9 in, 1 out]
                n389 = Unbundle(w639) -> (w636:string[])
                n390 = Match First String(2:w636, 3:w640) -> (0:w635:i32)  [unwired: 1 out]
                n391 = property on="Test Ring" class="Ring (strict)"("Value"=w635, "Strings []"=w636) -> ()  [unwired: 2 in, 2 out]
                n392 = property on="Test Ring" class="Ring (strict)"("Visible"=TRUE) -> ()  [unwired: 2 in, 2 out]
                n393 = property on="Test Slider" class="Slide (strict)"("Visible"=FALSE) -> ()  [unwired: 2 in, 2 out]
              }
              frame "Exposure  **" {
                n394 = Index Array(array=w647, index=2) -> (element=w648:cluster{string[]})
                n395 = call <vilib>:"NT Read String.vi"("Name"=w650) -> ("String"=w649:string)  [unwired: 9 in, 1 out]
                n396 = Unbundle(w648) -> (w644:string[])
                n397 = Match First String(2:w644, 3:w649) -> (0:w645:i32)  [unwired: 1 out]
                n398 = property on="Test Ring" class="Ring (strict)"("Value"=w645, "Strings []"=w644) -> ()  [unwired: 2 in, 2 out]
                n399 = property on="Test Ring" class="Ring (strict)"("Visible"=TRUE) -> ()  [unwired: 2 in, 2 out]
                n400 = property on="Test Slider" class="Slide (strict)"("Visible"=FALSE) -> ()  [unwired: 2 in, 2 out]
              }
              frame "Exposure Priority  **" {
                n401 = Index Array(array=w656, index=3) -> (element=w657:cluster{string[]})
                n402 = call <vilib>:"NT Read String.vi"("Name"=w659) -> ("String"=w658:string)  [unwired: 9 in, 1 out]
                n403 = Unbundle(w657) -> (w653:string[])
                n404 = Match First String(2:w653, 3:w658) -> (0:w654:i32)  [unwired: 1 out]
                n405 = property on="Test Ring" class="Ring (strict)"("Value"=w654, "Strings []"=w653) -> ()  [unwired: 2 in, 2 out]
                n406 = property on="Test Ring" class="Ring (strict)"("Visible"=TRUE) -> ()  [unwired: 2 in, 2 out]
                n407 = property on="Test Slider" class="Slide (strict)"("Visible"=FALSE) -> ()  [unwired: 2 in, 2 out]
              }
              frame "Color Enable  **" {
                n408 = Index Array(array=w665, index=4) -> (element=w666:cluster{string[]})
                n409 = call <vilib>:"NT Read String.vi"("Name"=w668) -> ("String"=w667:string)  [unwired: 9 in, 1 out]
                n410 = Unbundle(w666) -> (w662:string[])
                n411 = Match First String(2:w662, 3:w667) -> (0:w663:i32)  [unwired: 1 out]
                n412 = property on="Test Ring" class="Ring (strict)"("Value"=w663, "Strings []"=w662) -> ()  [unwired: 2 in, 2 out]
                n413 = property on="Test Ring" class="Ring (strict)"("Visible"=TRUE) -> ()  [unwired: 2 in, 2 out]
                n414 = property on="Test Slider" class="Slide (strict)"("Visible"=FALSE) -> ()  [unwired: 2 in, 2 out]
              }
              frame Default {
                n415 = property on="Test Ring" class="Ring (strict)"("Visible"=FALSE) -> ()  [unwired: 2 in, 2 out]
                n416 = property on="Test Slider" class="Slide (strict)"("Visible"=FALSE) -> ()  [unwired: 2 in, 2 out]
              }
              frame "Brightness  **", "Color Level  **", "Compression  **", "FPS  **", "Sharpness  **" {
                n417 = call <vilib>:"NT Read Number.vi"("Name"=w674) -> ("Numeric"=w673:dbl)  [unwired: 9 in, 1 out]
                n418 = local write "Test Slider"(w673) -> ()
                n419 = property on="Test Slider" class="Slide (strict)"("Visible"=TRUE, "Scale.Maximum"=100.0 ("Scale.Range:Maximum")) -> ()  [unwired: 2 in, 2 out]
                n420 = property on="Test Ring" class="Ring (strict)"("Visible"=FALSE) -> ()  [unwired: 2 in, 2 out]
              }
            }
          }
        }
        n421 = property on="Progress" class="Clust (strict)"("Visible"=FALSE) -> ()  [unwired: 2 in, 2 out]
      }
      event "Test Name": Mouse Enter {
        # "Populate the ring with the list of tests"
        n422 = event-data() -> ()  [unwired: 1 in, 1 out]
        n423 = call <vilib>:"NT Read String Array.vi"("Name"="TestMode/TestList") -> ("String Array"=w682:string[])  [unwired: 9 in, 1 out]
        n424 = Build Array (concatenate)("Select the test to run...", w682) -> (w681:string[])
        n425 = property on="Test Name" class="Ring (strict)"("Strings []"=w681) -> ()  [unwired: 2 in, 2 out]
      }
      event "Test Name": Value Change {
        w684 = FALSE ("Visible")
        # "Tell the robot the test name to run"
        n426 = event-data() -> ("NewVal"=w688:u16)  [unwired: 1 in]
        n427 = property on="Test Name" class="Ring (strict)"() -> ("Strings []"=w689:string[])  [unwired: 2 in, 2 out]
        n428 = local write "Progress"(T6 {"Test Progress"=0, "Test Progress Text"=""} ("Progress")) -> ()
        n429 = Index Array(array=w689, index=w688) -> (element=w687:string)
        n430 = call <vilib>:"NT Write String.vi"("String"=w687, "Name"="TestMode/TestName") -> ()  [unwired: 9 in, 1 out]
        n431 = property on="Progress" class="Clust (strict)"("Visible"=TRUE) -> ()  [unwired: 2 in, 2 out]
        n432 = property on="Motor" class="Clust (strict)"("Visible"=w684) -> ()  [unwired: 2 in, 2 out]
        n433 = property on="Test Slider" class="Slide (strict)"("Visible"=w684) -> ()  [unwired: 2 in, 2 out]
        n434 = property on="On/Off" class="Bool (strict)"("Visible"=w684) -> ()  [unwired: 2 in, 2 out]
        n435 = property on="Rev/Fwd" class="Clust (strict)"("Visible"=w684) -> ()  [unwired: 2 in, 2 out]
        n436 = property on="Test Ring" class="Ring (strict)"("Visible"=w684) -> ()  [unwired: 2 in, 2 out]
      }
      event "Select Auto": Mouse Enter {
        # "Populate the combo box with the list of autonomous options"
        n437 = event-data() -> ()  [unwired: 1 in, 1 out]
        n438 = call <vilib>:"NT Read String Array.vi"("Name"="Auto List") -> ("String Array"=w691:string[])  [unwired: 9 in, 1 out]
        n439 = property on="Select Auto" class="CmbBox"("Strings[]"=w691) -> ()  [unwired: 2 in, 2 out]
      }
      event "Select Auto": Value Change {
        # "User modified the Auto Selection. Write to NT variable so robot knows."
        n440 = event-data() -> ("NewVal"=w694:string)  [unwired: 1 in]
        n441 = call <vilib>:"NT Write String.vi"("String"=w694, "Name"="Auto Selector") -> ()  [unwired: 9 in, 1 out]
      }
      event "Command Selection": Value Change {
        # "Get the params and show in table"
        n442 = event-data() -> ("NewVal"=w700:i32)  [unwired: 1 in]
        n443 = property on="Command Selection" class="MCListbox (strict)"() -> ("ItemNames"=w698:string[][])  [unwired: 2 in, 2 out]
        n444 = call <vilib>:"WPI_DashboardUpdate Command Params.vi"("NewVal"=w700, "Commands"=w698, "Param Tbl"=w699) -> ()  [unwired: 8 in, 1 out]
      }
      event "Execute Command": Value Change {
        # "Started one, Unique ID holds\nresponse"
        n445 = event-data() -> ()  [unwired: 1 in, 1 out]
        n446 = property on="Command Selection" class="MCListbox (strict)"() -> ("ItemNames"=w711:string[][])  [unwired: 2 in, 2 out]
        n447 = Index Array(array=w711, index (row)="Command Selection", index (col)=0) -> (element=w709:string)
        n448 = call <vilib>:"Invoke Commands.vi"("Command Params"="Command Params", "Function Name"=w709) -> ("Params"=w705:u8, "Started"=w704:bool)  [unwired: 7 in, 1 out]
        n449 = Array Subset(array="Command Params", length (row)=w705) -> (w706:string[][])  [unwired: 3 in]
        n450 = Select(t="Executing" ("Cmd Status"), s=w704, f="" ("Cmd Status")) -> (s? t:f=→"Cmd Status":string)
      }
      event "Command Selection": Double Click {
        n451 = event-data() -> ("Row"=w719:i32)  [unwired: 1 in]
        n452 = property on="Command Selection" class="MCListbox (strict)"() -> ("ItemNames"=w722:string[][])  [unwired: 2 in, 2 out]
        n453 = local read "Command Params"() -> (w718:string[][])
        n454 = Index Array(array=w722, index (row)=w719, index (col)=0) -> (element=w720:string)
        n455 = call <vilib>:"Invoke Commands.vi"("Command Params"=w718, "Function Name"=w720) -> ("Params"=w717:u8, "Started"=w712:bool)  [unwired: 7 in, 1 out]
        n456 = Array Subset(array=w718, length (row)=w717) -> (w716:string[][])  [unwired: 3 in]
        n457 = Select(t="Executing" ("Cmd Status"), s=w712, f="" ("Cmd Status")) -> (s? t:f=w713:string)
        n458 = local write "Cmd Status"(w713) -> ()
      }
      event "CheckList": Double Click {
        # "Shift clears all"
        # "Update symbols on the listbox"
        n459 = event-data() -> ("PlatMods.Shift"=w724:bool, "Row"=w726:i32)  [unwired: 1 in]
        n460 = case shown="True" w724 {
          tunnel: w726 -> [w730 _]
          tunnel: 1 -> [w729 _]
          frame False {
            n461 = property on="CheckList" class="LstBox (strict)"() -> ("Item Symbols"=w728:i32[])  [unwired: 2 in, 2 out]
            n462 = Replace Array Subset(array=w728, new element=w729, index=w730) -> (w727:i32[])
            n463 = property on="CheckList" class="LstBox (strict)"("Item Symbols"=w727) -> ()  [unwired: 2 in, 2 out]
          }
          frame True {
            w731 = 0 ("Top Row")
            n464 = property on="CheckList" class="LstBox (strict)"() -> ("Number of Rows"=w733:u32)  [unwired: 2 in, 2 out]
            n465 = Initialize Array(0, w733) -> (w732:i32[])
            n466 = property on="CheckList" class="LstBox (strict)"("Top Row"=w731, "Value"=w731, "Item Symbols"=w732) -> ()  [unwired: 2 in, 2 out]
          }
        }
      }
      event "CheckList": Key Down {
        # "Update symbols on the listbox\nLeft and right keys check and uncheck"
        n467 = event-data() -> ("VKey"=w737:T21)  [unwired: 1 in]
        n468 = case shown="\"Left\", \"Right\"" w737 {
          selector: w737 -> [w742 _]
          tunnel: eventvkey."Left" ("VKey") -> [w740 _]
          frame "Left", "Right" {
            n469 = Equal?(x=w740, y=w742) -> (x = y?=w741:bool)
            n470 = Select(t=0, s=w741, f=1) -> (s? t:f=w743:i32)
            n471 = property on="CheckList" class="LstBox (strict)"() -> ("Item Symbols"=w746:i32[])  [unwired: 2 in, 2 out]
            n472 = Replace Array Subset(array=w746, new element=w743, index="CheckList") -> (w745:i32[])
            n473 = property on="CheckList" class="LstBox (strict)"("Item Symbols"=w745) -> ()  [unwired: 2 in, 2 out]
          }
          frame Default {
          }
        }
      }
      event "Motor.Enable": Value Change {
        # "When the test mode otor enable helper is set, update that\ntree row item's value"
        n474 = event-data() -> ("NewVal"=w752:bool)  [unwired: 1 in]
        n475 = Unbundle("Motor") -> ("Value"=w751:dbl)  [unwired: 1 out]
        n476 = Select(t=w751, s=w752, f=0.0) -> (s? t:f=w749:dbl)
        n477 = call <vilib>:"NT Write Number.vi"("Numeric"=w749, "Name"=w748) -> ()  [unwired: 9 in, 1 out]
      }
      event "Test Slider": Value Change {
        # "When the test mode slider helper is set, update that\ntree row item's value"
        n478 = event-data() -> ("NewVal"=w755:dbl)  [unwired: 1 in]
        n479 = call <vilib>:"NT Write Number.vi"("Numeric"=w755, "Name"=w756) -> ()  [unwired: 9 in, 1 out]
      }
      event "On/Off": Value Change {
        # "When the test mode on/off helper value is set, update that\ntree row item's value"
        n480 = event-data() -> ("NewVal"=w760:bool)  [unwired: 1 in]
        n481 = Boolean To (0,1)(Boolean=w760) -> (0, 1=w759:i16)
        n482 = call <vilib>:"NT Write Number.vi"("Numeric"=w759, "Name"=w758) -> ()  [unwired: 9 in, 1 out]
      }
      event "Rev/Fwd": Value Change {
        # "When the test mode helper value for relays is set, update that\ntree row item's value"
        n483 = event-data() -> ("NewVal.Forward"=w768:bool, "NewVal.Reverse"=w767:bool)  [unwired: 1 in]
        n484 = Boolean To (0,1)(Boolean=w768) -> (0, 1=w764:i16)
        n485 = Boolean To (0,1)(Boolean=w767) -> (0, 1=w766:i16)
        n486 = Negate(x=w766) -> (-x=w765:i16)
        n487 = Add(x=w764, y=w765) -> (x+y=w763:i16)
        n488 = call <vilib>:"NT Write Number.vi"("Numeric"=w763, "Name"=w762) -> ()  [unwired: 9 in, 1 out]
      }
      event "Test Ring": Value Change {
        # "When a test mode helper value is selected from the ring,\nset the tree item's variable to the string value"
        n489 = event-data() -> ("NewVal"=w772:u16)  [unwired: 1 in]
        n490 = property on="Test Ring" class="Ring (strict)"() -> ("Strings []"=w773:string[])  [unwired: 2 in, 2 out]
        n491 = Index Array(array=w773, index=w772) -> (element=w771:string)
        n492 = call <vilib>:"NT Write String.vi"("String"=w771, "Name"=w770) -> ()  [unwired: 9 in, 1 out]
      }
      event "Rec Mode": Value Change {
        # "Update globals for recording mode and path to read log from.\nClear when logging and let NetworkTables set path for vision to\nuse."
        n493 = event-data() -> ("NewVal"=w784:enum32{"Stop", "Record", "Playback"})  [unwired: 1 in]
        n494 = global write "WPI_DashboardLogging Global.vi" "Logging Filename"(path "") -> ()
        n495 = global write "WPI_DashboardLogging Global.vi" "Recording"(w784) -> ()
        n496 = case shown="\"Playback\"" w784 {
          tunnel: w783 -> [_ w786 w795]
          tunnel: [_ _ w794] -> w781
          tunnel: [_ _ w793] -> _
          tunnel: w779 -> [_ _ w791]
          tunnel: cluster{i32, i32} {-250, 170} -> [_ _ w790]
          tunnel: [_ _ T22 {"Image Size"=TRUE, "Image Type"=TRUE, "Pixel Value"=TRUE, "ROI Information"=TRUE, "Zoom Factor"=FALSE} ("Image Information Shown:All Elements")] -> w774
          tunnel: [_ _ TRUE ("Zoom Factor")] -> w775
          tunnel: w777 -> [_ _ w787]
          frame Default {
          }
          frame "Stop", "Record" {
            # "Place Window too"
            n497 = invoke class="VI" method="FP.Close"(reference=w786) -> (reference out=w785:refnum<vi>)  [unwired: 2 in, 2 out]
            n498 = invoke class="VI" method="Abort VI"(reference=w785) -> ()  [unwired: 2 in, 3 out]
          }
          frame "Playback" {
            n499 = call "Open Playback Panel.vi"("Offset"=w790, "DB VI Ref"=w791, "Playback in"=w795) -> ("Playback out"=w792:refnum<vi>)  [unwired: 8 in]
            n500 = register-events(w792, w787) -> (reference out=w794:refnum<event-registration>, error out=w793:errorcluster)  [unwired: 2 in]
          }
        }
        n501 = property on="Camera Image Right" class="ImageControl"("Image Information Shown"=w774, "Image Information Visible"=w775) -> ()  [unwired: 2 in, 2 out]
        n502 = property on="Camera Image1" class="ImageControl"("Image Information Shown"=w774, "Image Information Visible"=w775) -> ()  [unwired: 2 in, 2 out]
        n503 = call <vilib>:"WPI_DashboardNT Log FieldName Cache.vi"("Operation"=enum16{"Lookup/Add", "Index", "Clear"}."Clear") -> ()  [unwired: 8 in, 3 out]
      }
      event Panel Close {
        w797 = enum32{"Stop", "Record", "Playback"}."Stop" ("Rec Mode")
        # "Playback window has been closed, abort"
        n504 = event-data() -> ()  [unwired: 1 in, 4 out]
        n505 = local write "Rec Mode"(w797) -> ()
        n506 = global write "WPI_DashboardLogging Global.vi" "Recording"(w797) -> ()
      }
      event Panel Close {
        # "Abort playback window and ourself"
        n507 = event-data() -> ()  [unwired: 1 in, 4 out]
        n508 = invoke class="VI" method="FP.Close"(reference=w801) -> (reference out=w800:refnum<vi>)  [unwired: 2 in, 2 out]
        n509 = invoke class="VI" method="Abort VI"(reference=w800) -> (error out=w799:errorcluster)  [unwired: 2 in, 2 out]
        n510 = invoke class="VI" method="Abort VI"(error in=w799) -> ()  [unwired: 2 in, 3 out]
      }
      event User Event {
        n511 = event-data() -> ("IDs"=w808:cluster{"RPC field ID":u16, "Unique ID":u16}, "String"=w807:string)  [unwired: 1 in]
        n512 = Bundle("IDs"=w808, "String"=w807) -> (w806:T10)  [unwired: 1 in]
        n513 = call <vilib>:"Retrieve RPC Response.vi"("RPC Response"=w806) -> ("Output"=w804:string[][])  [unwired: 10 in]
        n514 = Build Array (concatenate)(w802, w804) -> (w803:string[][])
        n515 = local write "Command Params"(w803) -> ()
        n516 = local write "Cmd Status"("" ("Cmd Status")) -> ()
      }
      event "Tree": Double Click {
        n517 = event-data() -> ("PlatMods"=w814:T25, "Tag"=w811:string)  [unwired: 1 in]
        n518 = Unbundle(w814) -> ("Shift"=w813:bool)  [unwired: 4 out]
        n519 = String Subset(string=w811, length (rest)=1 ("length (rest)")) -> (substring=w810:string)  [unwired: 1 in]
        n520 = Not(x=w813) -> (.not. x?=w812:bool)
        n521 = case shown="\"/\"" w810 {
          tunnel: w811 -> [_ w817]
          tunnel: w812 -> [_ w816]
          frame Default {
          }
          frame "/" {
            n522 = call <vilib>:"NT Update Persistence.vi"("Persistence"=w816, "Name"=w817) -> ()  [unwired: 9 in, 1 out]
          }
        }
      }
    }
  }
  n523 = while {
    tunnel: w66 -> [w819]
    i -> [w822]
    stop <- FALSE stop-if-true
    n524 = Wait (ms)(milliseconds to wait=u32 100) -> ()  [unwired: 1 out]
    n525 = case shown="\"Playback\"" "Rec Mode" {
      tunnel: w822 -> [_ _ w837]
      tunnel: [u32 2829099 ("Base Color") u32 11141120 ("Target Color") w826] -> w818
      frame "Stop", Default {
        # "Reset the color, extra updates don't cost much"
      }
      frame "Record" {
      }
      frame "Playback" {
        # "Playback"
        n526 = Quotient & Remainder(x=w837, y=u32 50 ("milliseconds to wait")) -> (x-y*floor(x/y)=w833:u32)  [unwired: 1 out]
        n527 = Divide(x=w833, y=u32 50 ("milliseconds to wait")) -> (x/y=w830:dbl)
        n528 = Multiply(x=6.283185307179586, y=w830) -> (x*y=w835:dbl)
        n529 = Sine(x=w835) -> (sin(x)=w834:dbl)
        n530 = Absolute Value(x=w834) -> (abs(x)=w827:dbl)
        n531 = call "Interpolate RGB Color.vi"("Proportion"=w827, "Target Color"=u32 30976, "Base Color"=u32 2829099) -> ("Result Color"=w826:u32)  [unwired: 8 in]
      }
    }
    n532 = property class="Pane"(reference=w819, "PaneColor"=w818) -> ()  [unwired: 1 in, 2 out]
  }
  n533 = local write "Dashboard Tab"(T3."TeleOp" ("Dashboard Tab")) -> ()
  n534 = while {
    tunnel: u16 1741 ("timeout ms (25000)") -> [w839]
    stop <- FALSE stop-if-true
    n535 = TCP Create Listener(10:w839) -> (0:w838:errorcluster, 3:w840:refnum<k5>)  [unwired: 4 in, 1 out]
    n536 = case shown="No Error" w838 {
      selector: w838 -> [w842 _]
      tunnel: w840 -> [w843 _]
      frame No Error {
        n537 = while {
          tunnel: w843 -> [w846]
          tunnel: w842 -> [w845]
          stop <- FALSE stop-if-true
          n538 = TCP Wait On Listener(8:w845, 11:w846) -> (0:w847:errorcluster, 4:w848:refnum<k5>)  [unwired: 2 in, 3 out]
          n539 = local write "TCP"(w848) -> ()
          n540 = case shown="No Error" w847 {
            frame No Error {
            }
            frame Error {
              n541 = Wait (ms)(milliseconds to wait=u32 1000) -> ()  [unwired: 1 out]
            }
          }
        }
      }
      frame Error {
        n542 = Wait (ms)(milliseconds to wait=u32 1000) -> ()  [unwired: 1 out]
      }
    }
  }
  n543 = while {
    shift-right: [w866] -> _
    shift-left: _ -> [w919]
    shift-right: [w870] -> _
    shift-left: _ -> [w909]
    stop <- FALSE stop-if-true
    n544 = control-ref of="Ret_CARGO Left"() -> (w875:refnum<vi>)
    n545 = control-ref of="Ret_CARGO Right"() -> (w874:refnum<vi>)
    n546 = control-ref of="Ret_HATCH Left"() -> (w860:refnum<vi>)
    n547 = control-ref of="Ret_HATCH Right"() -> (w859:refnum<vi>)
    n548 = control-ref of="Ret_CARGO Center"() -> (w856:refnum<vi>)
    n549 = To Long Integer(number="Reticule") -> (32bit integer=w900:i32)
    n550 = First Call?() -> (First Call?: T/F=w883:bool)
    n551 = Multiply(x=w900, y=2) -> (x*y=w899:i32)
    n552 = Increment(x=w899) -> (x+1=w878:i32)
    n553 = case shown="True" w883 {
      tunnel: w875 -> [_ w940]
      tunnel: [w924 w937] -> w866
      tunnel: w919 -> [w924 _]
      tunnel: w874 -> [_ w934]
      tunnel: w860 -> [_ w933]
      tunnel: w859 -> [_ w932]
      tunnel: w856 -> [_ w927]
      frame False {
      }
      frame True {
        n554 = property class="Bool (strict)"(reference=w927) -> ("Left"=w926:i32, "Top"=w925:i32)  [unwired: 1 in, 2 out]
        n555 = property class="Bool (strict)"(reference=w940) -> ("Left"=w939:i32, "Top"=w938:i32)  [unwired: 1 in, 2 out]
        n556 = property class="Bool (strict)"(reference=w933) -> ("Left"=w931:i32, "Top"=w930:i32)  [unwired: 1 in, 2 out]
        n557 = property class="Bool (strict)"(reference=w932) -> ("Left"=w929:i32, "Top"=w928:i32)  [unwired: 1 in, 2 out]
        n558 = property class="Bool (strict)"(reference=w934) -> ("Left"=w936:i32, "Top"=w935:i32)  [unwired: 1 in, 2 out]
        n559 = Build Array(w939, w938, w936, w935, w931, w930, w929, w928, w926, w925) -> (w937:i32[])
      }
    }
    n560 = Bundle("Ret_CARGO Left"=w875, "Ret_CARGO Right"=w874, "Ret_HATCH Left"=w860, "Ret_HATCH Right"=w859, "Ret_CARGO Center"=w856) -> (w868:T26)  [unwired: 1 in]
    n561 = Index Array(array=w909, index #1=w899, index #2=w878) -> (element #1=w903:i32, element #2=w911:i32)
    n562 = Or(x="Up", y="Down") -> (x .or. y?=w915:bool)
    n563 = Or(x="Left", y="Right") -> (x .or. y?=w905:bool)
    n564 = Decrement(x=w911) -> (x-1=w918:i32)
    n565 = Increment(x=w911) -> (x+1=w917:i32)
    n566 = Decrement(x=w903) -> (x-1=w908:i32)
    n567 = Increment(x=w903) -> (x+1=w907:i32)
    n568 = Select(t=w918, s="Up", f=w917) -> (s? t:f=w916:i32)
    n569 = Select(t=w908, s="Left", f=w907) -> (s? t:f=w906:i32)
    n570 = Select(t=w916, s=w915, f=w911) -> (s? t:f=w877:i32)
    n571 = Select(t=w906, s=w905, f=w903) -> (s? t:f=w904:i32)
    n572 = Replace Array Subset(array=w909, new element #1=w904, index #1=w899, new element #2=w877, index #2=w878) -> (w876:i32[])
    n573 = Current VI's Path() -> (path=w891:path)
    n574 = Strip Path(path=w891) -> (stripped path=w890:path)  [unwired: 1 out]
    n575 = Strip Path(path=w890) -> (stripped path=w889:path)  [unwired: 1 out]
    n576 = Cluster To Array(cluster=w868) -> (array=w873:refnum<vi>[])
    n577 = Build Path(base path=w889, name or relative path=path "reticule positions.txt" ("XML File Path")) -> (appended path=w888:path)
    n578 = Array Size(array=w873) -> (size(s)=w869:i32)
    n579 = call-poly <vilib>:"Read From XML File.vi"("XML File Path"=w888) -> ("XML Elements"=w887:string[])  [unwired: 8 in, 2 out]
    n580 = Multiply(x=2 ("dimension size"), y=w869) -> (x*y=w882:i32)
    n581 = Initialize Array(0, w882) -> (w852:i32[])
    n582 = Index Array(array=w887, index=0) -> (element=w885:string)
    n583 = Unflatten From XML(xml string=w885, type=w852) -> (value=w851:i32[])  [unwired: 1 in, 1 out]
    n584 = First Call?() -> (First Call?: T/F=w910:bool)
    n585 = Select(t=w851, s=w910, f=w876) -> (s? t:f=w870:i32[])
    n586 = Add(x=w870, y=w866) -> (x+y=w867:i32[])
    n587 = Unbundle(w868) -> ("Ret_CARGO Left"=w872:refnum<vi>, "Ret_CARGO Right"=w871:refnum<vi>, "Ret_HATCH Left"=w858:refnum<vi>, "Ret_HATCH Right"=w857:refnum<vi>, "Ret_CARGO Center"=w855:refnum<vi>)
    n588 = Index Array(array=w867, index #1=0 ("index")) -> (element #1=w897:i32, element #2=w896:i32, element #3=w880:i32, element #4=w879:i32, element #5=w864:i32, element #6=w863:i32, element #7=w862:i32, element #8=w861:i32, element #9=w854:i32, element #10=w853:i32)  [unwired: 9 in]
    n589 = Flatten To XML(anything=w870) -> (xml string=w895:string)
    n590 = call "RisingEdgeTrigger.vi"("Raw Signal"="Save") -> ("Trigger"=w894:bool)
    n591 = property class="Bool (strict)"(reference=w872, "Left"=w897, "Top"=w896) -> ()  [unwired: 1 in, 2 out]
    n592 = property class="Bool (strict)"(reference=w871, "Left"=w880, "Top"=w879) -> ()  [unwired: 1 in, 2 out]
    n593 = property class="Bool (strict)"(reference=w857, "Left"=w862, "Top"=w861) -> ()  [unwired: 1 in, 2 out]
    n594 = property class="Bool (strict)"(reference=w855, "Left"=w854, "Top"=w853) -> ()  [unwired: 1 in, 2 out]
    n595 = property class="Bool (strict)"(reference=w858, "Left"=w864, "Top"=w863) -> ()  [unwired: 1 in, 2 out]
    n596 = case shown="True" w894 {
      tunnel: w895 -> [_ w923]
      tunnel: w888 -> [_ w922]
      frame False {
      }
      frame True {
        n597 = call-poly <vilib>:"Write to XML File.vi"("XML Input"=w923, "XML File Path"=w922) -> ()  [unwired: 7 in, 3 out]
      }
    }
    n598 = Wait (ms)(milliseconds to wait=u32 100) -> ()  [unwired: 1 out]
  }
  n599 = property on="On/Off" class="Bool (strict)"("Visible"=w37) -> ()  [unwired: 2 in, 2 out]
  n600 = property on="Motor" class="Clust (strict)"("Visible"=w37) -> ()  [unwired: 2 in, 2 out]
  n601 = property on="Progress" class="Clust (strict)"("Visible"=w37) -> ()  [unwired: 2 in, 2 out]
  n602 = property on="Test Ring" class="Ring (strict)"("Visible"=w37) -> ()  [unwired: 2 in, 2 out]
  n603 = property on="Rev/Fwd" class="Clust (strict)"("Visible"=w37) -> ()  [unwired: 2 in, 2 out]
  n604 = local write "Command Selection"(u16 0 ("milliseconds to wait")) -> ()
  n605 = local write "Command Params"(string[][] [] ("Command Params")) -> ()
  n606 = global write "WPI_DashboardLogging Global.vi" "Recording"(w60) -> ()
  n607 = local write "Rec Mode"(w60) -> ()
  n608 = call <vilib>:"NT Write String.vi"("String"="Select Auto", "Name"="Auto Selector") -> ()  [unwired: 9 in, 1 out]
  n609 = while {
    stop <- FALSE stop-if-true
    n610 = local read "Master_Caution"() -> (w943:bool)
    n611 = case shown="True" w943 {
      frame False {
      }
      frame True {
        n612 = call <vilib>:"Beep.vi"("duration (msec)"=u32 1000) -> ()  [unwired: 11 in]
        n613 = Wait (ms)(milliseconds to wait=u32 1000) -> ()  [unwired: 1 out]
      }
    }
    n614 = Wait (ms)(milliseconds to wait=u32 100) -> ()  [unwired: 1 out]
  }
